vi "1_2_VisualAD_Train_Eval_Investigate.vi"(0 "NNFE_Paths":T1={"CFG"=path "D:/Ngene/GitHub/deepltk_examples/3_Image_Processing/36_Anomaly_Detection/NNFE/WRN_50_2_2_L3/WRN_50_2_2_BBoneL3.cfg", "BIN"=path "D:/Ngene/GitHub/deepltk_examples/3_Image_Processing/36_Anomaly_Detection/NNFE/WRN_50_2_2_L3/WRN_50_2_2_BBoneL3.bin"}, 1 "Dest. Path":path=path "D:/working", 2 "Dataset_Path(Train)":path=path "D:/Ngene/GitHub/deepltk_examples/3_Image_Processing/36_Anomaly_Detection/Dataset/Cards_3OfSpades/train", 3 "Dataset_Path(Validation)":path=path "D:/Ngene/GitHub/deepltk_examples/3_Image_Processing/36_Anomaly_Detection/Dataset/Cards_3OfSpades/test", 4 "Ground_Truth_Folder_Path":path, 5 "error in":errorcluster, 6 "NNFE CFG":T7={"Name"="3OfSpades", "Layer_Selection_By"=enum."Stride", "Feature_Layers"={"[LayerID, PatchSize]"=[{"Layer_ID"=4, "Patch_Size"=3}, {"Layer_ID"=16, "Patch_Size"=5}]}, "Interpolation_Type"=enum."Bi-Linear"}, 7 "Dim_Reduction":T11={"Method"=enum."Rnd_Proj", "Target_Dim"=300, "Seed"=42}, 8 "NNPC_Setup":T2={"Input_Dims"={"C"=3, "H"=320, "W"=272}, "mBatch"=1, "Device"=enum."GPU", "GPU Id"=0}, 9 "CoreSet_Params":T5={"Distance_Metric"=enum."Euclidean", "CoreSet_Size"=10000.0, "Start_idx"=3}) -> (11 "MemBank Size":i32=10000, 13 "dT_Total":dbl=8.99153380000007 format="%.2f", 14 "Model Paths":T1={"CFG"=path "D:/working/NNPC_3OfSpades.cfg", "BIN"=path "D:/working/NNPC_3OfSpades.bin"}, 15 "Evaluation Metrics":T13={"Evaluation_Metrics(Pixel)"={"Scores(Good)"={"X Values"=[2.1673927682638165, 2.522966259121895, 2.8785397499799728, 3.2341132408380506, 3.589686731696129, 3.945260222554207, 4.300833713412285, 4.656407204270362, 5.011980695128441, 5.367554185986519, 5.723127676844596, 6.078701167702675, 6.434274658560753, 6.78984814941883, 7.145421640276909, 7.500995131134987, 7.856568621993065, 8.212142112851144, 8.567715603709221, 8.923289094567298, 9.278862585425376, 9.634436076283453, 9.990009567141533, 10.345583057999612, 10.70115654885769, 11.056730039715767, 11.412303530573844, 11.767877021431921, 12.12345051229, 12.479024003148078, 12.834597494006157, 13.190170984864235, 13.545744475722312, 13.90131796658039, 14.256891457438469, 14.612464948296546, 14.968038439154626, 15.323611930012703, 15.67918542087078, 16.034758911728858, 16.390332402586935, 16.745905893445013, 17.10147938430309, 17.457052875161168, 17.81262636601925, 18.168199856877326, 18.523773347735403, 18.879346838593484, 19.234920329451562, 19.59049382030964, 19.946067311167717, 20.301640802025794, 20.65721429288387, 21.01278778374195, 21.368361274600026, 21.723934765458107, 22.079508256316185, 22.435081747174262, 22.79065523803234, 23.146228728890417, 23.501802219748498, 23.857375710606576, 24.212949201464653, 24.56852269232273, 24.924096183180808, 25.279669674038885, 25.635243164896963, 25.99081665575504, 26.34639014661312, 26.7019636374712, 27.057537128329276, 27.413110619187353, 27.76868411004543, 28.124257600903512, 28.47983109176159, 28.835404582619667, 29.190978073477744, 29.54655156433582, 29.9021250551939, 30.257698546051977, 30.613272036910054, 30.968845527768135, 31.324419018626212, 31.67999250948429, 32.035566000342364, 32.39113949120044, 32.746712982058526, 33.1022864729166, 33.45785996377468, 33.81343345463276, 34.169006945490835, 34.52458043634891, 34.88015392720699, 35.23572741806507, 35.591300908923145, 35.94687439978122, 36.30244789063931, 36.658021381497385, 37.01359487235546, 37.36916836321354], "Histogram: h(x)"=[1, 13, 52, 84, 115, 188, 266, 742, 1993, 4173, 6263, 6873, 6767, 7084, 7294, 7385, 7892, 8253, 8640, 10003, 11295, 15100, 22306, 35779, 62043, 98920, 135969, 166467, 171557, 159572, 143358, 124535, 97728, 76352, 57016, 39265, 26147, 16432, 10767, 6225, 3406, 1671, 480, 165, 84, 0, 0, 0, 0, 0, 0, 0, 0, 0, 0, 0, 0, 0, 0, 0, 0, 0, 0, 0, 0, 0, 0, 0, 0, 0, 0, 0, 0, 0, 0, 0, 0, 0, 0, 0, 0, 0, 0, 0, 0, 0, 0, 0, 0, 0, 0, 0, 0, 0, 0, 0, 0, 0, 0, 0]}, "Scores(Bad)"={"X Values"=[2.1673927682638165, 2.522966259121895, 2.8785397499799728, 3.2341132408380506, 3.589686731696129, 3.945260222554207, 4.300833713412285, 4.656407204270362, 5.011980695128441, 5.367554185986519, 5.723127676844596, 6.078701167702675, 6.434274658560753, 6.78984814941883, 7.145421640276909, 7.500995131134987, 7.856568621993065, 8.212142112851144, 8.567715603709221, 8.923289094567298, 9.278862585425376, 9.634436076283453, 9.990009567141533, 10.345583057999612, 10.70115654885769, 11.056730039715767, 11.412303530573844, 11.767877021431921, 12.12345051229, 12.479024003148078, 12.834597494006157, 13.190170984864235, 13.545744475722312, 13.90131796658039, 14.256891457438469, 14.612464948296546, 14.968038439154626, 15.323611930012703, 15.67918542087078, 16.034758911728858, 16.390332402586935, 16.745905893445013, 17.10147938430309, 17.457052875161168, 17.81262636601925, 18.168199856877326, 18.523773347735403, 18.879346838593484, 19.234920329451562, 19.59049382030964, 19.946067311167717, 20.301640802025794, 20.65721429288387, 21.01278778374195, 21.368361274600026, 21.723934765458107, 22.079508256316185, 22.435081747174262, 22.79065523803234, 23.146228728890417, 23.501802219748498, 23.857375710606576, 24.212949201464653, 24.56852269232273, 24.924096183180808, 25.279669674038885, 25.635243164896963, 25.99081665575504, 26.34639014661312, 26.7019636374712, 27.057537128329276, 27.413110619187353, 27.76868411004543, 28.124257600903512, 28.47983109176159, 28.835404582619667, 29.190978073477744, 29.54655156433582, 29.9021250551939, 30.257698546051977, 30.613272036910054, 30.968845527768135, 31.324419018626212, 31.67999250948429, 32.035566000342364, 32.39113949120044, 32.746712982058526, 33.1022864729166, 33.45785996377468, 33.81343345463276, 34.169006945490835, 34.52458043634891, 34.88015392720699, 35.23572741806507, 35.591300908923145, 35.94687439978122, 36.30244789063931, 36.658021381497385, 37.01359487235546, 37.36916836321354], "Histogram: h(x)"=[8, 31, 105, 130, 214, 331, 610, 1315, 3212, 6453, 8836, 10903, 11627, 10731, 11893, 12681, 12586, 13151, 14679, 16111, 18152, 22770, 29905, 42923, 63976, 97131, 135040, 170047, 186000, 191189, 185809, 165467, 145942, 127004, 108579, 95369, 82034, 66973, 56446, 48734, 41993, 35860, 33251, 29363, 25936, 23587, 20606, 18581, 16403, 14613, 12756, 11558, 10975, 10578, 9887, 8831, 9074, 8615, 7970, 7376, 6857, 6950, 6755, 6391, 5609, 4681, 3976, 3457, 3231, 2862, 2517, 2294, 2141, 1977, 1864, 1796, 1866, 1798, 1579, 1481, 1246, 1074, 1034, 809, 645, 542, 391, 316, 340, 331, 318, 257, 219, 149, 152, 115, 99, 73, 53, 45]}, "Eval Stats"={"Scores(Good)"={"Min"=2.329183, "Max"=17.973423}, "Scores(Bad)"={"Min"=1.989606, "Max"=37.546955}, "# of Samples(Good)"=1566720, "# of Samples(Bad)"=2611200, "AUROC"=-1.0, "F1_Max"=-1.0, "Thrshld(F1_Max)"=17.973423, "Prec.(F1_Max)"=-1.0, "Recall(F1_Max)"=-1.0, "FPR(F1_Max)"=-1.0, "FNR(F1_Max)"=-1.0}}, "Evaluation_Metrics(Image)"={"Scores(Good)"={"X Values"=[16.63672716140747, 16.8714089012146, 17.10609064102173, 17.34077238082886, 17.575454120635985, 17.810135860443115, 18.044817600250244, 18.279499340057374, 18.514181079864503, 18.74886281967163, 18.98354455947876, 19.218226299285888, 19.452908039093018, 19.687589778900147, 19.922271518707277, 20.156953258514406, 20.391634998321535, 20.62631673812866, 20.86099847793579, 21.09568021774292, 21.33036195755005, 21.565043697357176, 21.799725437164305, 22.034407176971435, 22.269088916778564, 22.503770656585694, 22.738452396392823, 22.973134136199953, 23.207815876007082, 23.44249761581421, 23.677179355621337, 23.911861095428467, 24.146542835235596, 24.381224575042726, 24.615906314849852, 24.85058805465698, 25.08526979446411, 25.31995153427124, 25.55463327407837, 25.7893150138855, 26.02399675369263, 26.258678493499758, 26.493360233306888, 26.728041973114017, 26.962723712921143, 27.197405452728272, 27.4320871925354, 27.666768932342528, 27.901450672149657, 28.136132411956787, 28.370814151763916, 28.605495891571046, 28.840177631378175, 29.074859371185305, 29.309541110992434, 29.544222850799564, 29.77890459060669, 30.01358633041382, 30.24826807022095, 30.482949810028074, 30.717631549835204, 30.952313289642333, 31.186995029449463, 31.421676769256592, 31.656358509063722, 31.89104024887085, 32.12572198867798, 32.36040372848511, 32.59508546829224, 32.82976720809936, 33.06444894790649, 33.29913068771362, 33.53381242752075, 33.76849416732788, 34.00317590713501, 34.23785764694214, 34.47253938674927, 34.7072211265564, 34.94190286636353, 35.17658460617066, 35.411266345977786, 35.645948085784916, 35.880629825592045, 36.115311565399175, 36.349993305206304, 36.584675045013434, 36.819356784820556, 37.054038524627686, 37.288720264434815, 37.523402004241944, 37.758083744049074, 37.9927654838562, 38.22744722366333, 38.462128963470455, 38.696810703277585, 38.931492443084714, 39.166174182891844, 39.40085592269897, 39.6355376625061, 39.87021940231323], "Histogram: h(x)"=[2, 0, 0, 1, 2, 0, 1, 2, 3, 3, 2, 1, 0, 0, 1, 0, 0, 0, 0, 0, 0, 0, 0, 0, 0, 0, 0, 0, 0, 0, 0, 0, 0, 0, 0, 0, 0, 0, 0, 0, 0, 0, 0, 0, 0, 0, 0, 0, 0, 0, 0, 0, 0, 0, 0, 0, 0, 0, 0, 0, 0, 0, 0, 0, 0, 0, 0, 0, 0, 0, 0, 0, 0, 0, 0, 0, 0, 0, 0, 0, 0, 0, 0, 0, 0, 0, 0, 0, 0, 0, 0, 0, 0, 0, 0, 0, 0, 0, 0, 0]}, "Scores(Bad)"={"X Values"=[16.63672716140747, 16.8714089012146, 17.10609064102173, 17.34077238082886, 17.575454120635985, 17.810135860443115, 18.044817600250244, 18.279499340057374, 18.514181079864503, 18.74886281967163, 18.98354455947876, 19.218226299285888, 19.452908039093018, 19.687589778900147, 19.922271518707277, 20.156953258514406, 20.391634998321535, 20.62631673812866, 20.86099847793579, 21.09568021774292, 21.33036195755005, 21.565043697357176, 21.799725437164305, 22.034407176971435, 22.269088916778564, 22.503770656585694, 22.738452396392823, 22.973134136199953, 23.207815876007082, 23.44249761581421, 23.677179355621337, 23.911861095428467, 24.146542835235596, 24.381224575042726, 24.615906314849852, 24.85058805465698, 25.08526979446411, 25.31995153427124, 25.55463327407837, 25.7893150138855, 26.02399675369263, 26.258678493499758, 26.493360233306888, 26.728041973114017, 26.962723712921143, 27.197405452728272, 27.4320871925354, 27.666768932342528, 27.901450672149657, 28.136132411956787, 28.370814151763916, 28.605495891571046, 28.840177631378175, 29.074859371185305, 29.309541110992434, 29.544222850799564, 29.77890459060669, 30.01358633041382, 30.24826807022095, 30.482949810028074, 30.717631549835204, 30.952313289642333, 31.186995029449463, 31.421676769256592, 31.656358509063722, 31.89104024887085, 32.12572198867798, 32.36040372848511, 32.59508546829224, 32.82976720809936, 33.06444894790649, 33.29913068771362, 33.53381242752075, 33.76849416732788, 34.00317590713501, 34.23785764694214, 34.47253938674927, 34.7072211265564, 34.94190286636353, 35.17658460617066, 35.411266345977786, 35.645948085784916, 35.880629825592045, 36.115311565399175, 36.349993305206304, 36.584675045013434, 36.819356784820556, 37.054038524627686, 37.288720264434815, 37.523402004241944, 37.758083744049074, 37.9927654838562, 38.22744722366333, 38.462128963470455, 38.696810703277585, 38.931492443084714, 39.166174182891844, 39.40085592269897, 39.6355376625061, 39.87021940231323], "Histogram: h(x)"=[0, 0, 0, 0, 0, 0, 0, 0, 0, 0, 0, 0, 0, 0, 0, 0, 0, 0, 0, 0, 0, 1, 0, 0, 0, 1, 0, 0, 0, 0, 0, 1, 0, 0, 0, 0, 0, 0, 1, 0, 0, 1, 0, 0, 0, 0, 1, 0, 1, 0, 2, 2, 0, 0, 0, 1, 1, 1, 1, 0, 2, 2, 0, 0, 0, 0, 2, 0, 0, 1, 0, 0, 1, 1, 0, 0, 0, 0, 0, 0, 0, 1, 0, 0, 0, 0, 0, 0, 1, 0, 0, 0, 0, 0, 2, 1, 0, 0, 0, 1]}, "Eval Stats"={"Scores(Good)"={"Min"=16.519386, "Max"=19.817144}, "Scores(Bad)"={"Min"=21.46867, "Max"=39.98756}, "# of Samples(Good)"=18, "# of Samples(Bad)"=30, "AUROC"=1.0904129, "F1_Max"=-1.0, "Thrshld(F1_Max)"=20.642906, "Prec.(F1_Max)"=-1.0, "Recall(F1_Max)"=-1.0, "FPR(F1_Max)"=-1.0, "FNR(F1_Max)"=-1.0}}} {"Evaluation_Metrics(Image)"."Eval Stats"."Recall(F1_Max)" format="%#.5f"; "Evaluation_Metrics(Image)"."Eval Stats"."FPR(F1_Max)" format="%#.5f"; "Evaluation_Metrics(Image)"."Eval Stats"."FNR(F1_Max)" format="%#.5f"; "Evaluation_Metrics(Image)"."Eval Stats"."Prec.(F1_Max)" format="%#.5f"; "Evaluation_Metrics(Image)"."Eval Stats"."F1_Max" format="%#.5f"; "Evaluation_Metrics(Image)"."Eval Stats"."AUROC" format="%#.5f"; "Evaluation_Metrics(Image)"."Eval Stats"."Scores(Bad)"."Min" format="%#_5g"; "Evaluation_Metrics(Image)"."Eval Stats"."Scores(Good)"."Min" format="%#_5g"; "Evaluation_Metrics(Image)"."Eval Stats"."Thrshld(F1_Max)" format="%#_5f"; "Evaluation_Metrics(Pixel)"."Eval Stats"."Recall(F1_Max)" format="%#.5f"; "Evaluation_Metrics(Pixel)"."Eval Stats"."FPR(F1_Max)" format="%#.5f"; "Evaluation_Metrics(Pixel)"."Eval Stats"."FNR(F1_Max)" format="%#.5f"; "Evaluation_Metrics(Pixel)"."Eval Stats"."Prec.(F1_Max)" format="%#.5f"; "Evaluation_Metrics(Pixel)"."Eval Stats"."F1_Max" format="%#.5f"; "Evaluation_Metrics(Pixel)"."Eval Stats"."AUROC" format="%#.5f"; "Evaluation_Metrics(Pixel)"."Eval Stats"."Scores(Bad)"."Min" format="%#_5g"; "Evaluation_Metrics(Pixel)"."Eval Stats"."Scores(Good)"."Min" format="%#_5g"; "Evaluation_Metrics(Pixel)"."Eval Stats"."Thrshld(F1_Max)" format="%#_5f"}, 18 "Dataset Size":i32=20)   [LabVIEW 2020]
uses:
  <vilib>/Ngene/DeepLTK Anomaly Detection Addon/Toolkit/API/Controls/NN_Paths.ctl
  <vilib>/Ngene/DeepLTK Anomaly Detection Addon/Toolkit/API/Controls/NNPC_Setup.ctl
  <vilib>/Ngene/Deep Learning Toolkit/Toolkit/NN_Data/API/NN_Dims(C,H,W).ctl
  <vilib>/Ngene/Deep Learning Toolkit/Toolkit/NN_Network/Controls/NN_Device.ctl
  <vilib>/Ngene/DeepLTK Anomaly Detection Addon/Toolkit/API/Controls/NNPC_Coreset_Params.ctl
  <vilib>/Ngene/DeepLTK Anomaly Detection Addon/Toolkit/API/Controls/Distance_Metric.ctl
  <vilib>/Ngene/DeepLTK Anomaly Detection Addon/Toolkit/API/Controls/NNFE_CFG.ctl
  <vilib>/Ngene/DeepLTK Anomaly Detection Addon/Toolkit/API/Controls/Layer_Selector.ctl
  <vilib>/Ngene/DeepLTK Anomaly Detection Addon/Toolkit/API/Controls/Feature_Layer_Selector.ctl
  <vilib>/Ngene/DeepLTK Anomaly Detection Addon/Toolkit/API/Controls/Interpolation_Selector.ctl
  <vilib>/Ngene/DeepLTK Anomaly Detection Addon/Toolkit/API/Controls/NNPC_Random_Projection_CFG.ctl
  <vilib>/Ngene/DeepLTK Anomaly Detection Addon/Toolkit/API/Controls/Dim_Reduction_Method.ctl
  <vilib>/Ngene/DeepLTK Anomaly Detection Addon/Toolkit/API/Controls/Evaluation_Metrics(Pixel_Image).ctl
  <vilib>/Ngene/DeepLTK Anomaly Detection Addon/Toolkit/API/Controls/Evaluation_Metrics.ctl
  <vilib>/Ngene/DeepLTK Anomaly Detection Addon/Toolkit/API/Controls/Eval_Results.ctl
  <vilib>/Ngene/DeepLTK Anomaly Detection Addon/Toolkit/API/Controls/MinMax.ctl
  subVIs/Feature_Retrieval/Controls/Patch_RF_Scales.ctl
  subVIs/Dataset_Reader/Controls/Read_Options.ctl
  <vilib>/Ngene/DeepLTK Anomaly Detection Addon/Toolkit/API/Controls/NNPC_PreProcessing_Options.ctl
  <vilib>/Ngene/DeepLTK Anomaly Detection Addon/Toolkit/API/Controls/Crop_CFG.ctl
  <vilib>/Ngene/DeepLTK Anomaly Detection Addon/Toolkit/API/Controls/NNPC_DS_Stats.ctl
  <vilib>/Ngene/DeepLTK Anomaly Detection Addon/Toolkit/API/Controls/Image_Stats_RGB.ctl
  subVIs/Train_Case_Investigation/Controls/Detection_Results.ctl
  <vilib>/Ngene/DeepLTK Anomaly Detection Addon/Toolkit/API/Controls/Feature_Scorer_Params.ctl
  <vilib>/Ngene/DeepLTK Anomaly Detection Addon/Toolkit/API/Controls/Gaussian_Blur.ctl
  <vilib>/vision/Image Controls.llb/IMAQ Image.ctl
  subVIs/Visualizer/Controls/Display_Options.ctl
  subVIs/Visualizer/Controls/ROI_Display_Options.ctl
  subVIs/Visualizer/Controls/Heatmap_Display_Options.ctl
  subVIs/Visualizer/Controls/ColorMap.ctl
  subVIs/Visualizer/Controls/Report_Images_CFG.ctl
  <vilib>/Ngene/CuLab - GPU Accelerated Toolkit/Toolkit/Low_Level/Tensor_Classes/T_Children/T2D/T2D_Children/T2D_SGL/T2D_SGL.lvclass
  subVIs/Feature_Retrieval/Controls/Dims(2D)ctl.ctl
  4cc6689b-300a-41eb-b37a-9ba3a5a9262f.vi
  f46c6ce4-2999-47cd-b61f-bf4da423de8f.vi
  <vilib>/Utility/High Resolution Relative Seconds.vi
  <vilib>/Ngene/DeepLTK Anomaly Detection Addon/Toolkit/API/NNPC_Predict/NNPC_Predict(Dataset).vi
  <vilib>/Ngene/DeepLTK Anomaly Detection Addon/Toolkit/API/NNPC_Predict/NNPC_Predict(Single).vi
  <vilib>/Ngene/Deep Learning Toolkit/Toolkit/NN_Data/subVIs/Get_Data_Vals/2D/NN_Data_Get_ValByRef(2D_SGL).vi
  <vilib>/Ngene/CuLab - GPU Accelerated Toolkit/Toolkit/Low_Level/Tensor_Classes/T_Children/T2D/T2D_Children/T2D_SGL/Pull.vi
  <vilib>/Ngene/DeepLTK Anomaly Detection Addon/Toolkit/DeepLTK_Anomaly_Detection_Addon.lvlib
  <vilib>/Ngene/Deep Learning Toolkit/Toolkit/Deep_Learning_Toolkit_by_Ngene.lvlib
  <vilib>/Ngene/CuLab - GPU Accelerated Toolkit/Toolkit/CuLab.lvlib
  <vilib>/ptbypt/NI_PtbyPt.lvlib
  <vilib>/vision/NI_Vision_Development_Module.lvlib
panel:
  out "Last Mouse Position:All Elements":cluster{"X":i32, "Y":i32}={"X"=128, "Y"=172}
  in  "?":enum32{"Train Eval", "Investigation"}(tab)
  out "dT_Gen_Embed":dbl=0.16472169999997277 format="%.2f"
  out "dT_Coreset":dbl=4.406857699999819 format="%.2f"
  out "Coreset_Max_Distances":sgl[](graph)
  out "dT_NN_Init":dbl=2.5163400999999794 format="%.2f"
  out "dT_Read_DS(Train)":dbl=0.30830639999976484 format="%.2f"
  out "dT_Read_DS(Test)":dbl=0.43927769999982047 format="%.2f"
  out "dT_Eval":dbl=0.9348227000000406 format="%.2f"
  out "dT_Predict(DS)":dbl=0.6623571000000084 format="%.2f"
  out "Coreset Max":sgl=72.34939
  out "Feature Size":i32=300
  out "Coreset Min":sgl=12.7185
  in  "Online_Coreset_Params":T5={"Distance_Metric"=enum."Euclidean", "CoreSet_Size"=-1.0, "Start_idx"=3}
  out "Closest_Train_Sample":T17(plugin-control)
  in  "UpScale Factor":sgl=1.0
  in  "index":i32=17 min=0 max=29
  out "Anomaly Detection Result":T17(plugin-control)
  out "Image_Thrshld (Eval)":sgl=20.6429
  in  "Image_Thrshld(Custom)":sgl=-1.0 format="%_5g"
  out "Pixel_Score(Max)":sgl=29.230766
  out "Image_File_Path":path=path "D:/Ngene/GitHub/deepltk_examples/3_Image_Processing/36_Anomaly_Detection/Dataset/Cards_3OfSpades/test/bad/bad_Cut_Twice_1967.bmp"
  out "Pixel_Thrshld (Eval)":sgl=17.9734
  out "Anomaly?":bool=TRUE
  out "Img_Score":sgl=30.951008
  in  "Pixel_Thrshld(Custom)":sgl=18.2 format="%_5g"
  in  "DS Selector":enum16{"Good", "Bad", "Both"}(ring)=enum."Bad"
  in  "Order":enum16{"Ascending", "Descending", "File"}(ring)
  out "error out":errorcluster
  in  "Closest_Idx":i32 min=0 max=3
  out "#Closest_Samples":i32=4
  in  "Feature Color":u32(colorbox)=2486016
  in  "ROI Scales":T18={"Receptive_Field"=1.0, "Patch"=1.0} {"Patch" min=0 max=0; "Receptive_Field" min=0 max=0}
  out "Closest_Score":sgl=15.526439
  in  "Show Patch Grid?":bool
  in  "Search Mode":bool
  in  "Heatmap Range":T16={"Min"=17.0, "Max"=19.0} {"Min" format="%#_5g"}
  in  "ROI Color":u32(colorbox)=16717824
  in  "Display_Image":T19(ring)=enum."HeatMap"
  out "dT_Predict":dbl=0.014165199999922606 format="%#_3p"
  in  "Stop":bool
  out "Closest_Train_File_Path":path=path "D:/Ngene/GitHub/deepltk_examples/3_Image_Processing/36_Anomaly_Detection/Dataset/Cards_3OfSpades/train/good_2169.bmp"
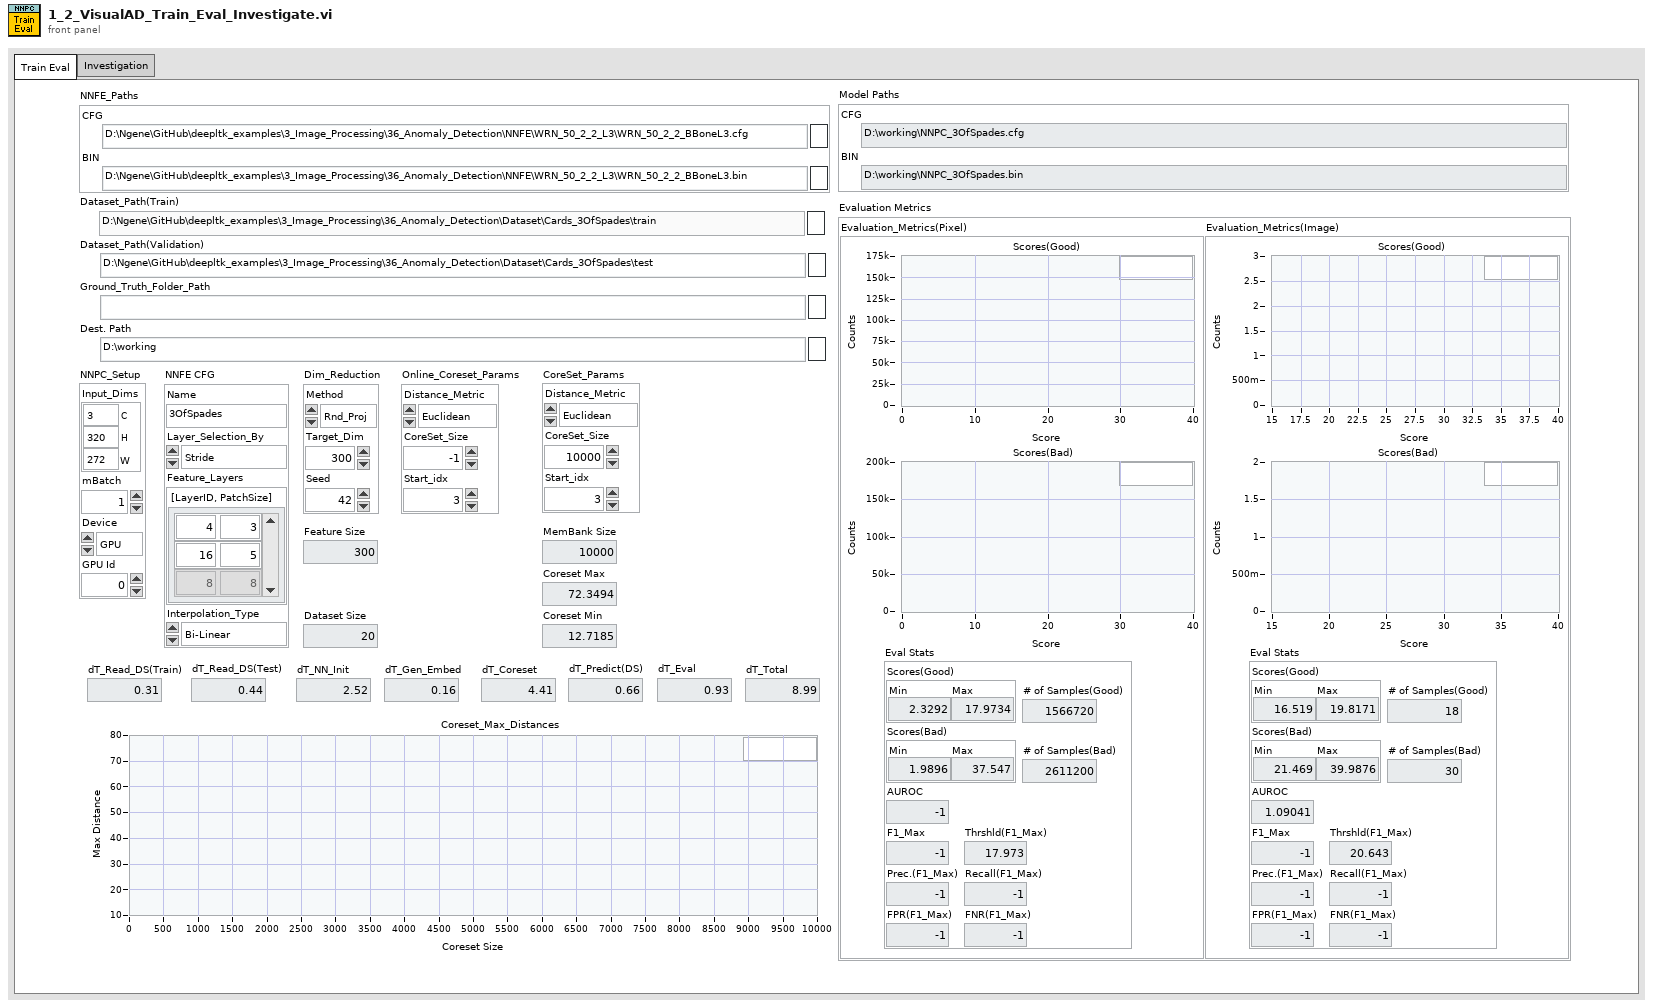
[diagram p1: front panel]
types:
  T1 = typedef "DeepLTK_Anomaly_Detection_Addon.lvlib/NN_Paths.ctl" = cluster{"CFG":path, "BIN":path}
  T2 = typedef "DeepLTK_Anomaly_Detection_Addon.lvlib/NNPC_Setup.ctl" = cluster{"Input_Dims":T3, "mBatch":i32, "Device":T4, "GPU Id":i32}
  T3 = typedef "Deep_Learning_Toolkit_by_Ngene.lvlib/NN_Dims(C,H,W).ctl" = cluster{"C":i32, "H":i32, "W":i32}
  T4 = typedef "Deep_Learning_Toolkit_by_Ngene.lvlib/NN_Device.ctl" = enum16{"CPU", "GPU"}
  T5 = typedef "DeepLTK_Anomaly_Detection_Addon.lvlib/NNPC_Coreset_Params.ctl" = cluster{"Distance_Metric":T6, "CoreSet_Size":sgl, "Start_idx":i32}
  T6 = typedef "DeepLTK_Anomaly_Detection_Addon.lvlib/Distance_Metric.ctl" = enum16{"Euclidean", "Cosine"}
  T7 = typedef "DeepLTK_Anomaly_Detection_Addon.lvlib/NNFE_CFG.ctl" = cluster{"Name":string, "Layer_Selection_By":T8, "Feature_Layers":T9, "Interpolation_Type":T10}
  T8 = typedef "DeepLTK_Anomaly_Detection_Addon.lvlib/Layer_Selector.ctl" = enum16{"Stride", "Layer_Idx"}
  T9 = typedef "DeepLTK_Anomaly_Detection_Addon.lvlib/Feature_Layer_Selector.ctl" = cluster{"[LayerID, PatchSize]":cluster{"Layer_ID":i32, "Patch_Size":i32}[]}
  T10 = typedef "DeepLTK_Anomaly_Detection_Addon.lvlib/Interpolation_Selector.ctl" = enum16{"Nearest", "Bi-Linear"}
  T11 = typedef "DeepLTK_Anomaly_Detection_Addon.lvlib/NNPC_Random_Projection_CFG.ctl" = cluster{"Method":T12, "Target_Dim":i32, "Seed":i32}
  T12 = typedef "DeepLTK_Anomaly_Detection_Addon.lvlib/Dim_Reduction_Method.ctl" = enum16{"None", "Rnd_Proj", "PCA"}
  T13 = typedef "DeepLTK_Anomaly_Detection_Addon.lvlib/Evaluation_Metrics(Pixel_Image).ctl" = cluster{"Evaluation_Metrics(Pixel)":T14, "Evaluation_Metrics(Image)":T14}
  T14 = typedef "DeepLTK_Anomaly_Detection_Addon.lvlib/Evaluation_Metrics.ctl" = cluster{"Scores(Good)":cluster{"X Values":dbl[], "Histogram: h(x)":i32[]}, "Scores(Bad)":cluster{"X Values":dbl[], "Histogram: h(x)":i32[]}, "Eval Stats":T15}
  T15 = typedef "DeepLTK_Anomaly_Detection_Addon.lvlib/Eval_Results.ctl" = cluster{"Scores(Good)":T16, "Scores(Bad)":T16, "# of Samples(Good)":i32, "# of Samples(Bad)":i32, "AUROC":sgl, "F1_Max":sgl, "Thrshld(F1_Max)":sgl, "Prec.(F1_Max)":sgl, "Recall(F1_Max)":sgl, "FPR(F1_Max)":sgl, "FNR(F1_Max)":sgl}
  T16 = typedef "DeepLTK_Anomaly_Detection_Addon.lvlib/MinMax.ctl" = cluster{"Min":sgl, "Max":sgl}
  T17 = typedef "IMAQ Image.ctl" = refnum<image>
  T18 = typedef "Patch_RF_Scales.ctl" = cluster{"Receptive_Field":sgl, "Patch":sgl}
  T19 = enum16{"Original", "Ground_Truth", "HeatMap", "Mask", "Segmentation"}
  T20 = typedef "Image Type" = u32
  T21 = typedef "DeepLTK_Anomaly_Detection_Addon.lvlib/Feature_Scorer_Params.ctl" = cluster{"Nearest_Neighbors":i32, "Calculate Anomaly Map":bool, "Gaussian_Blur":T22}
  T22 = typedef "DeepLTK_Anomaly_Detection_Addon.lvlib/Gaussian_Blur.ctl" = cluster{"Kernel_Size":i32, "Sigma":sgl}
  T23 = typedef "Detection_Results.ctl" = cluster{"Image Score":sgl, "Pixel Score":sgl[][], "File Path":path}
  T24 = typedef "Read_Options.ctl" = cluster{"Read Bads?":bool, "Read GTs?":bool, "Update. DS Stats?":bool}
  T25 = typedef "DeepLTK_Anomaly_Detection_Addon.lvlib/NNPC_PreProcessing_Options.ctl" = cluster{"DS_Name":string, "Input_Dims":T3, "Cropping":T26, "Interpolation Type":u32, "MultiStage_ReSample?":bool, "Dataset_Stats":T27}
  T26 = typedef "DeepLTK_Anomaly_Detection_Addon.lvlib/Crop_CFG.ctl" = cluster{"Left":sgl, "Top":sgl, "Right":sgl, "Bottom":sgl}
  T27 = typedef "DeepLTK_Anomaly_Detection_Addon.lvlib/NNPC_DS_Stats.ctl" = cluster{"means":T28, "stds":T28}
  T28 = typedef "DeepLTK_Anomaly_Detection_Addon.lvlib/Image_Stats_RGB.ctl" = cluster{"R":sgl, "G":sgl, "B":sgl}
  T29 = typedef "Deep_Learning_Toolkit_by_Ngene.lvlib/NN_DataSet(In3D_Out3D).ctl" = cluster{"Dataset_Size":i32, "Dims_In":T3, "Labels":string[], "File Paths":path[], "Outputs Ref.":T30, "Inputs Ref.":variant, "Dims_Out":T3, "Custom_Data":variant}
  T30 = typedef "Deep_Learning_Toolkit_by_Ngene.lvlib/NN_Data_ref(4D_SGL).ctl" = refnum<data-value>
  T31 = typedef "DeepLTK_Anomaly_Detection_Addon.lvlib/NNPC_Instance.ctl" = cluster{"Name":string, "NN":T32, "MemBank_Data":T46}
  T32 = typedef "Deep_Learning_Toolkit_by_Ngene.lvlib/NN.ctl" = cluster{"Name":string, "No of Layers":i32, "mBatch":i32, "Layers":T33[], "Dimty":T34, "Dims_In":T3, "Dims_Out":T3, "Working_Dir":path, "Train?":bool, "Train_Params":T35, "LR_Update_Policy":T38, "Session Data":T40, "Ground_truth":T41, "NNg_hdls":T42, "NN_Device":T4, "GPU Id":i32, "Labels":string[], "Loss_Type":T43, "Loss_Cfg_Prms":variant, "NNG_WS":T44, "DryRun?":bool}
  T33 = typedef "Deep_Learning_Toolkit_by_Ngene.lvlib/NN_Layer_ref.ctl" = refnum<file>
  T34 = typedef "Deep_Learning_Toolkit_by_Ngene.lvlib/NN_In_Out_Dim-ty.ctl" = enum8{"In1D_Out1D", "In3D_Out1D", "In3D_Out3D", "In3D_OutBBox"}
  T35 = typedef "Deep_Learning_Toolkit_by_Ngene.lvlib/NN_Train_Params.ctl" = cluster{"Optimizer":T36, "Beta_1":sgl, "Beta_2":sgl, "Weight Decay(L1)":sgl, "Weight Decay(L2)":sgl, "Data_Sampling":T37}
  T36 = typedef "Deep_Learning_Toolkit_by_Ngene.lvlib/NN_Train_Optimizer.ctl" = enum16{"SGD", "Adam", "Adagrad", "Adadelta", "RMSProp", "Nesterov"}
  T37 = typedef "Deep_Learning_Toolkit_by_Ngene.lvlib/NN_Train_Data_Sampling.ctl" = enum16{"Random", "Sequential"}
  T38 = typedef "Deep_Learning_Toolkit_by_Ngene.lvlib/NN_LR_Policy_Cfg.ctl" = cluster{"Policy_Type":T39, "LR0":dbl, "k":sgl, "WarmUp_Policy":enum16{"Step", "Ramp"}, "WarmUp_Iter":i32, "WarmUp_Ratio":sgl}
  T39 = typedef "Deep_Learning_Toolkit_by_Ngene.lvlib/NN_LR_Policy_Type.ctl" = enum16{"Manual", "Step", "Exp", "1/t"}
  T40 = typedef "Deep_Learning_Toolkit_by_Ngene.lvlib/NN_Train_Session_Data.ctl" = cluster{"Epochs":sgl, "Tot_Iter":i32, "LR":sgl, "LR_iter":i32}
  T41 = typedef "Deep_Learning_Toolkit_by_Ngene.lvlib/NN_Ground_truth.ctl" = cluster{"Y":variant}
  T42 = typedef "Deep_Learning_Toolkit_by_Ngene.lvlib/nng_cuda_handles.ctl" = cluster{"cudnn":u64, "cublas":u64, "stream":u64, "curand":u64}
  T43 = typedef "Deep_Learning_Toolkit_by_Ngene.lvlib/NN_Loss_Type.ctl" = enum16{"None", "MSE", "CrossEntropy", "YOLO_v2", "YOLO_v4"}
  T44 = typedef "Deep_Learning_Toolkit_by_Ngene.lvlib/NNG_WS.ctl" = cluster{"NNG_WS_Mem":T45, "Max_WS_Size":i64}
  T45 = typedef "Deep_Learning_Toolkit_by_Ngene.lvlib/NNg_WS_Mem_DVR.ctl" = refnum<data-value>
  T46 = typedef "DeepLTK_Anomaly_Detection_Addon.lvlib/MemBank_and_Norm_Variants.ctl" = cluster{"MemBank":variant, "MemBank Norm":variant}
  T47 = typedef "DeepLTK_Anomaly_Detection_Addon.lvlib/Feature_Coords(Idx,i,j).ctl" = cluster{"Idx":i32, "i":i32, "j":i32}
  T48 = typedef "imagedata.ctl" = cluster{"image type":i32, "image depth":i32, "image":u8[], "mask":u8[], "colors":u32[], "Rectangle":cluster{"left":i16, "top":i16, "right":i16, "bottom":i16}}
  T49 = typedef "DeepLTK_Anomaly_Detection_Addon.lvlib/NNPC_Evaluation_Results.ctl" = cluster{"Threshold(Image)":sgl, "Threshold(Pixel)":sgl, "Pixel_Range":cluster{"Min":sgl, "Max":sgl}}
  T50 = typedef "Selected_Coreset_Elements_and_Dim_Stride_Info.ctl" = cluster{"Dims_Out":T51, "Stride":i32, "Coreset_Elements":T47[]}
  T51 = typedef "Dims(2D)ctl.ctl" = cluster{"H":i32, "W":i32}
  T52 = typedef "Deep_Learning_Toolkit_by_Ngene.lvlib/NN_Layer.ctl" = cluster{"Name":string, "Layer_Data":T53, "Layer_Type":T54, "Dims_In":T3, "Layers_In":T33[], "Dims_Out":T3, "Layers_Out":T33[], "Metrics":T55, "GPU_Data":T56, "mBatch":i32, "NN_Device":T4, "NNg_hdls":T42, "Train?":bool, "Dimty":T57, "RecptField":T58, "Idx":i32}
  T53 = typedef "Deep_Learning_Toolkit_by_Ngene.lvlib/NN_Layer_Data_Refnum.ctl" = refnum<file>
  T54 = typedef "Deep_Learning_Toolkit_by_Ngene.lvlib/NN_Layer_Type.ctl" = enum16{"Input1D", "Input3D", "Conv1D", "Conv2D", "Conv2D_Adv", "MaxPool", "AvgPool", "UpSample", "DropOut3D", "ShortCut", "Concat", "SoftMax3D", "FC", "DropOut", "Softmax", "Flatten", "YOLO_v2", "YOLO_v4", "Activation", "BatchNormalization", "LayerNormalization", "Scale", "Unsupported"}
  T55 = typedef "Deep_Learning_Toolkit_by_Ngene.lvlib/NN_Layer_Metrics.ctl" = cluster{"Data":dbl, "Params":dbl, "Ops":dbl}
  T56 = typedef "Deep_Learning_Toolkit_by_Ngene.lvlib/NNg_Layer_Data_Refnum.ctl" = refnum<file>
  T57 = typedef "Deep_Learning_Toolkit_by_Ngene.lvlib/NN_Layer_Dimty.ctl" = enum16{"1D", "3D"}
  T58 = typedef "Deep_Learning_Toolkit_by_Ngene.lvlib/NN_Layer_RF_State.ctl" = cluster{"Dims":T59, "J":T59}
  T59 = typedef "Deep_Learning_Toolkit_by_Ngene.lvlib/NN_Dims(V,H).ctl" = cluster{"V":i32, "H":i32}
  T60 = typedef "Display_Options.ctl" = cluster{"ROI_Options":T61, "Heatmap_Options":T62, "Report_Images_CFG":T64}
  T61 = typedef "ROI_Display_Options.ctl" = cluster{"Color":u32, "Width":u32, "Drawing Mode":enum16{"Frame", "Fill"}}
  T62 = typedef "Heatmap_Display_Options.ctl" = cluster{"ColorMap":T63, "Alpha":sgl, "Heatmap Range":T16}
  T63 = typedef "ColorMap.ctl" = enum16{"Jet", "Perula", "Inferno", "Plasma", "Viridis"}
  T64 = typedef "Report_Images_CFG.ctl" = cluster{"Original Image":bool, "Ground Truth":bool, "HeatMap":bool, "Mask":bool, "Segmentation":bool}
  T65 = typedef "Anomaly_Detection_Results_Imgs.ctl" = cluster{"Image":T17, "Ground Truth":T17, "Predicted Heat Map":T17, "Predicted Mask":T17, "Segmentation":T17}
  T66 = typedef "Closest_Sample_Info.ctl" = cluster{"Score":sgl, "Feature_Coords":T47}
  T67 = typedef "Deep_Learning_Toolkit_by_Ngene.lvlib/NN_BBox.ctl" = cluster{"x":sgl, "y":sgl, "w":sgl, "h":sgl}
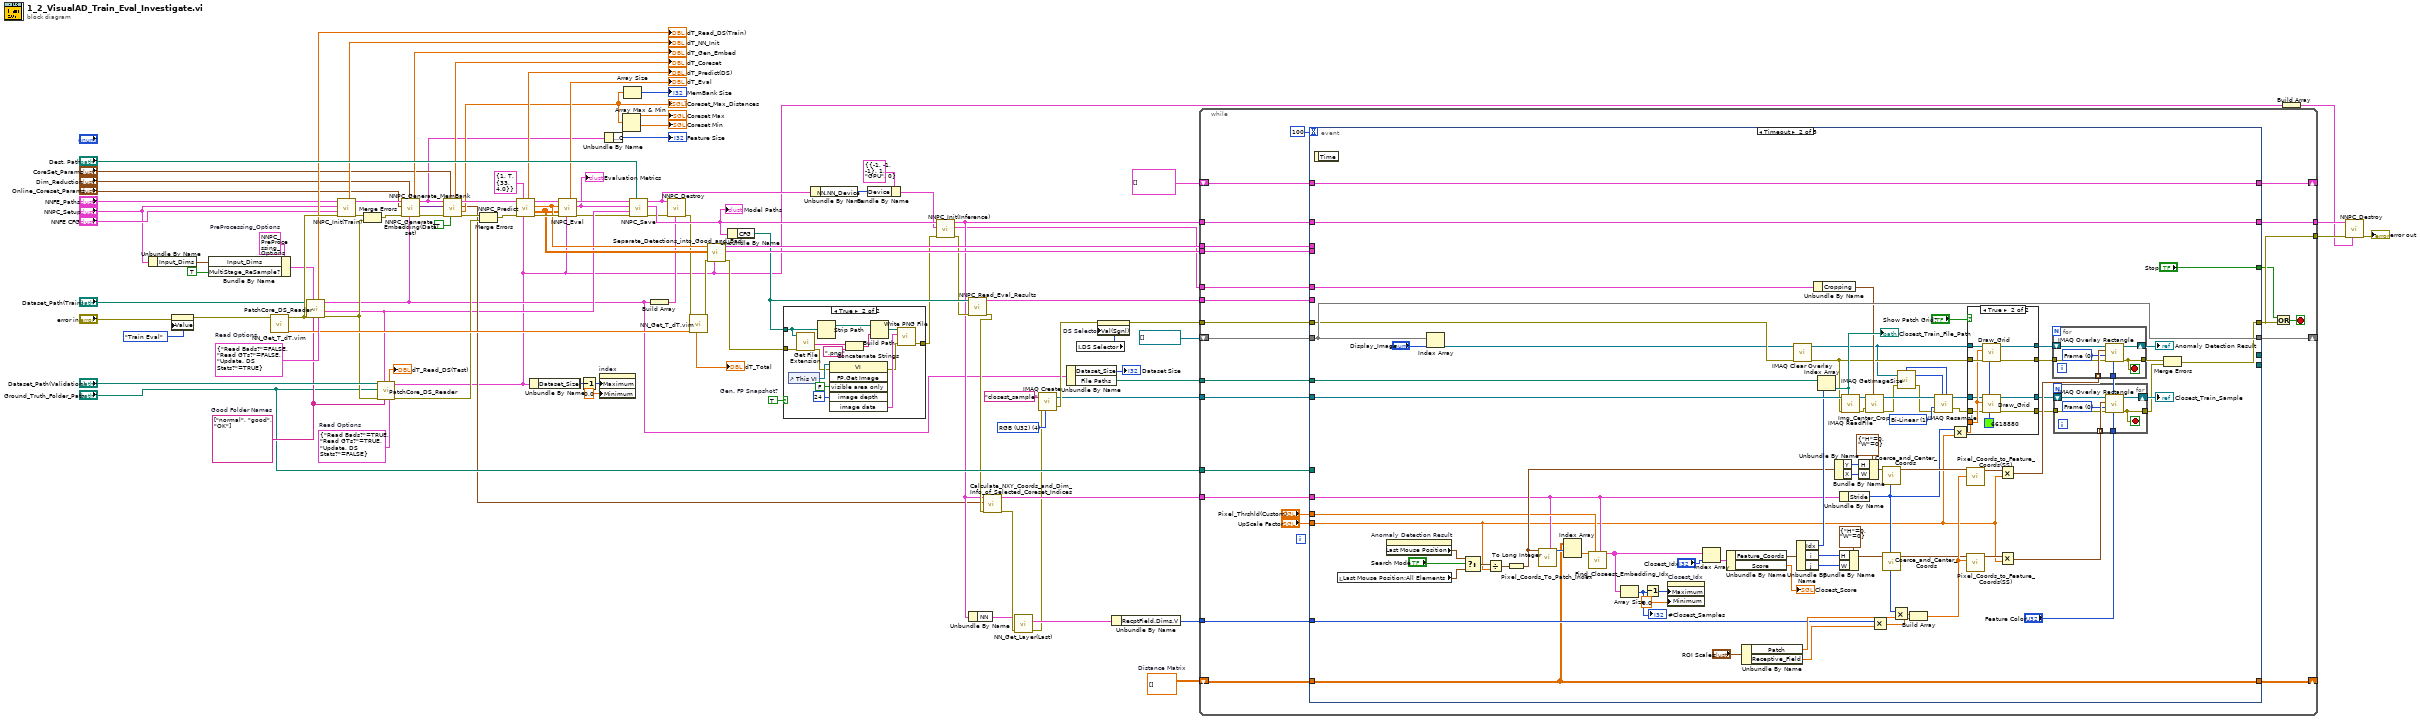
[diagram p0: block diagram]
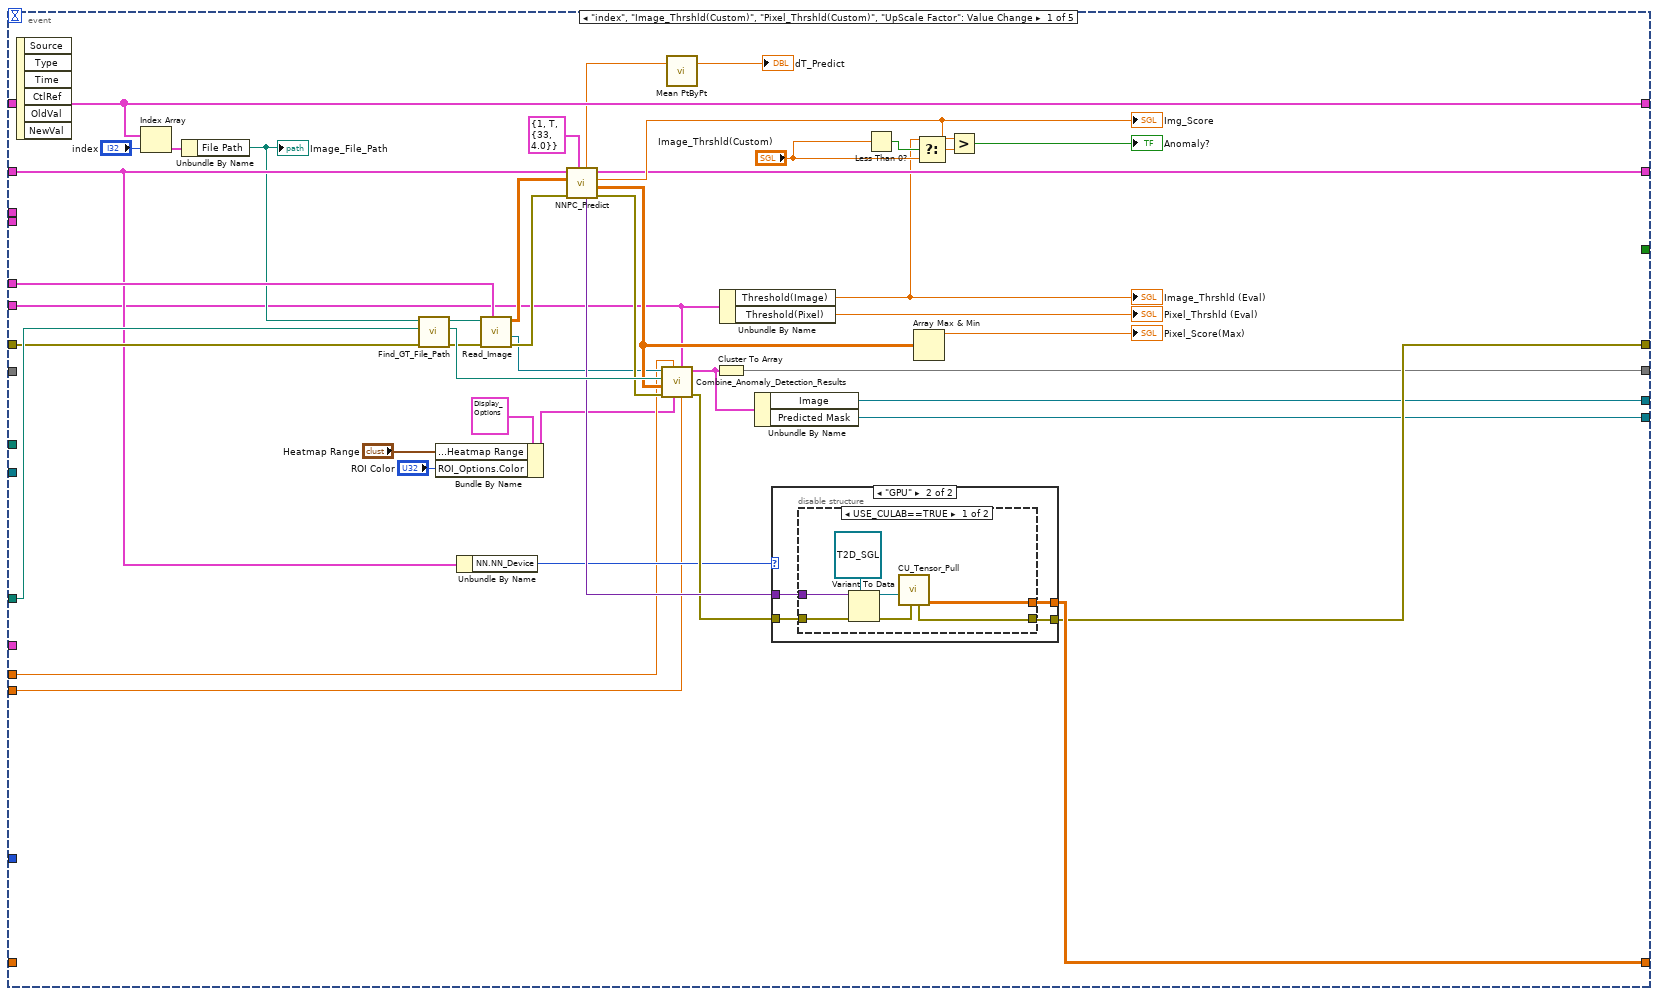
[diagram p2: hidden frame]
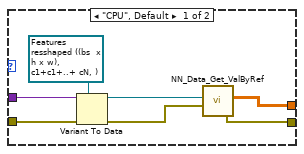
[diagram p3: hidden frame]
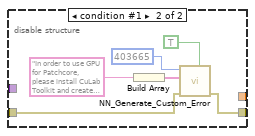
[diagram p4: hidden frame]
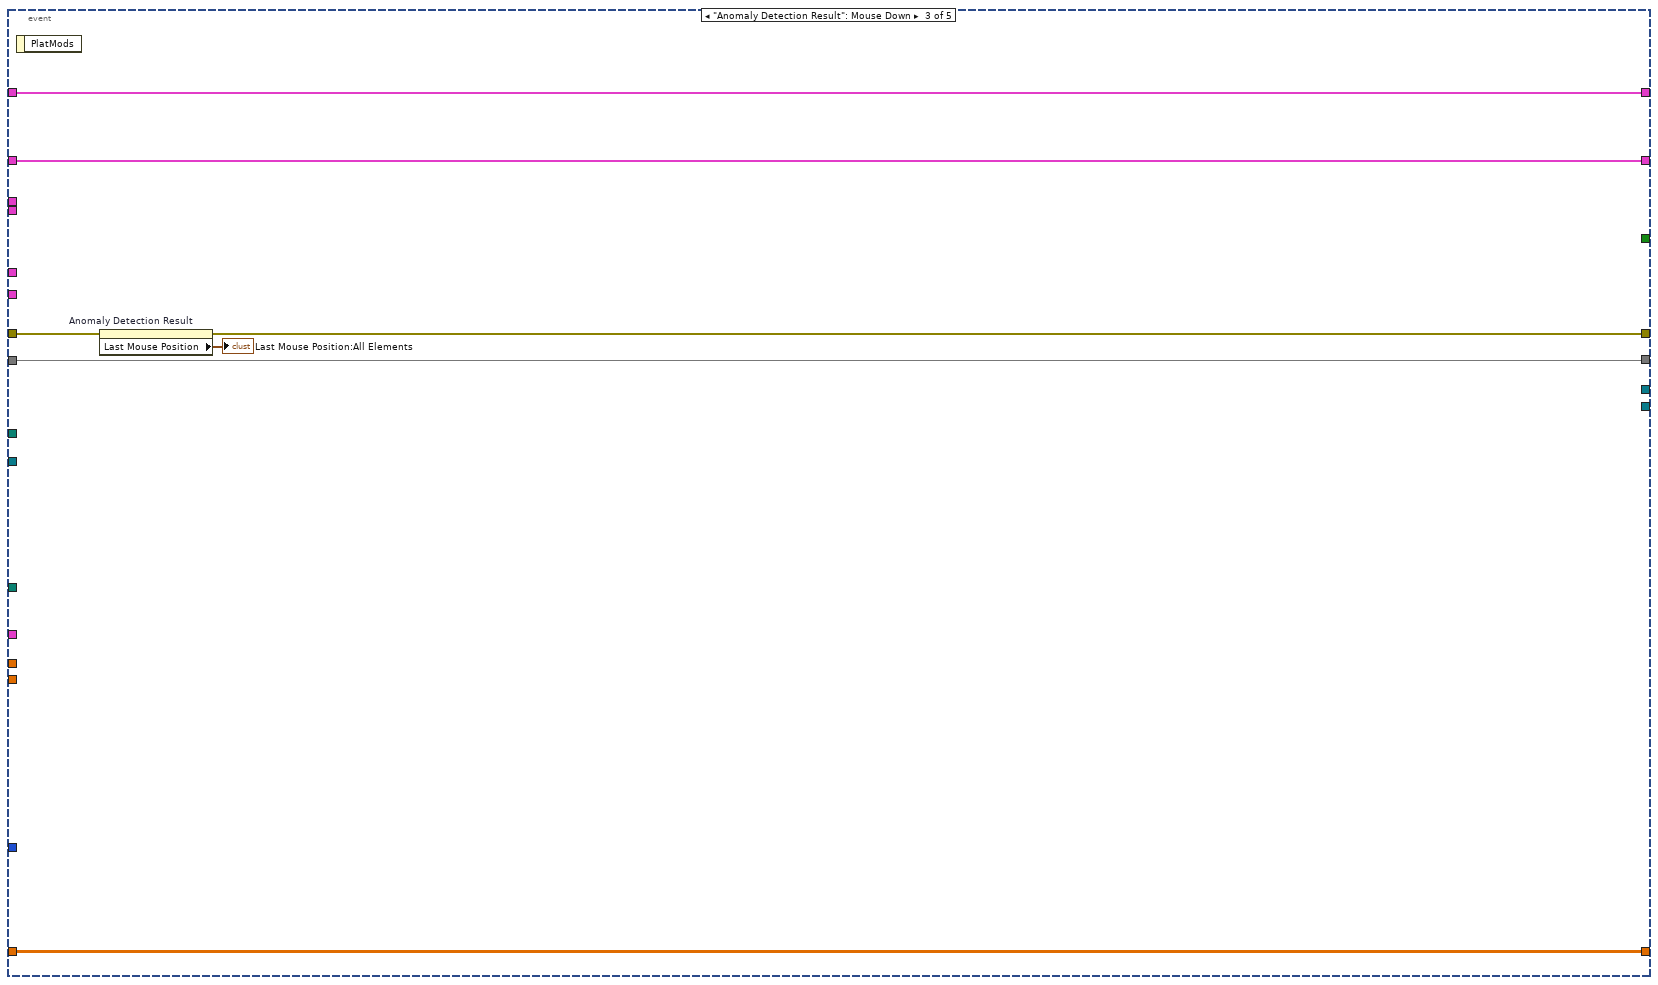
[diagram p6: hidden frame]
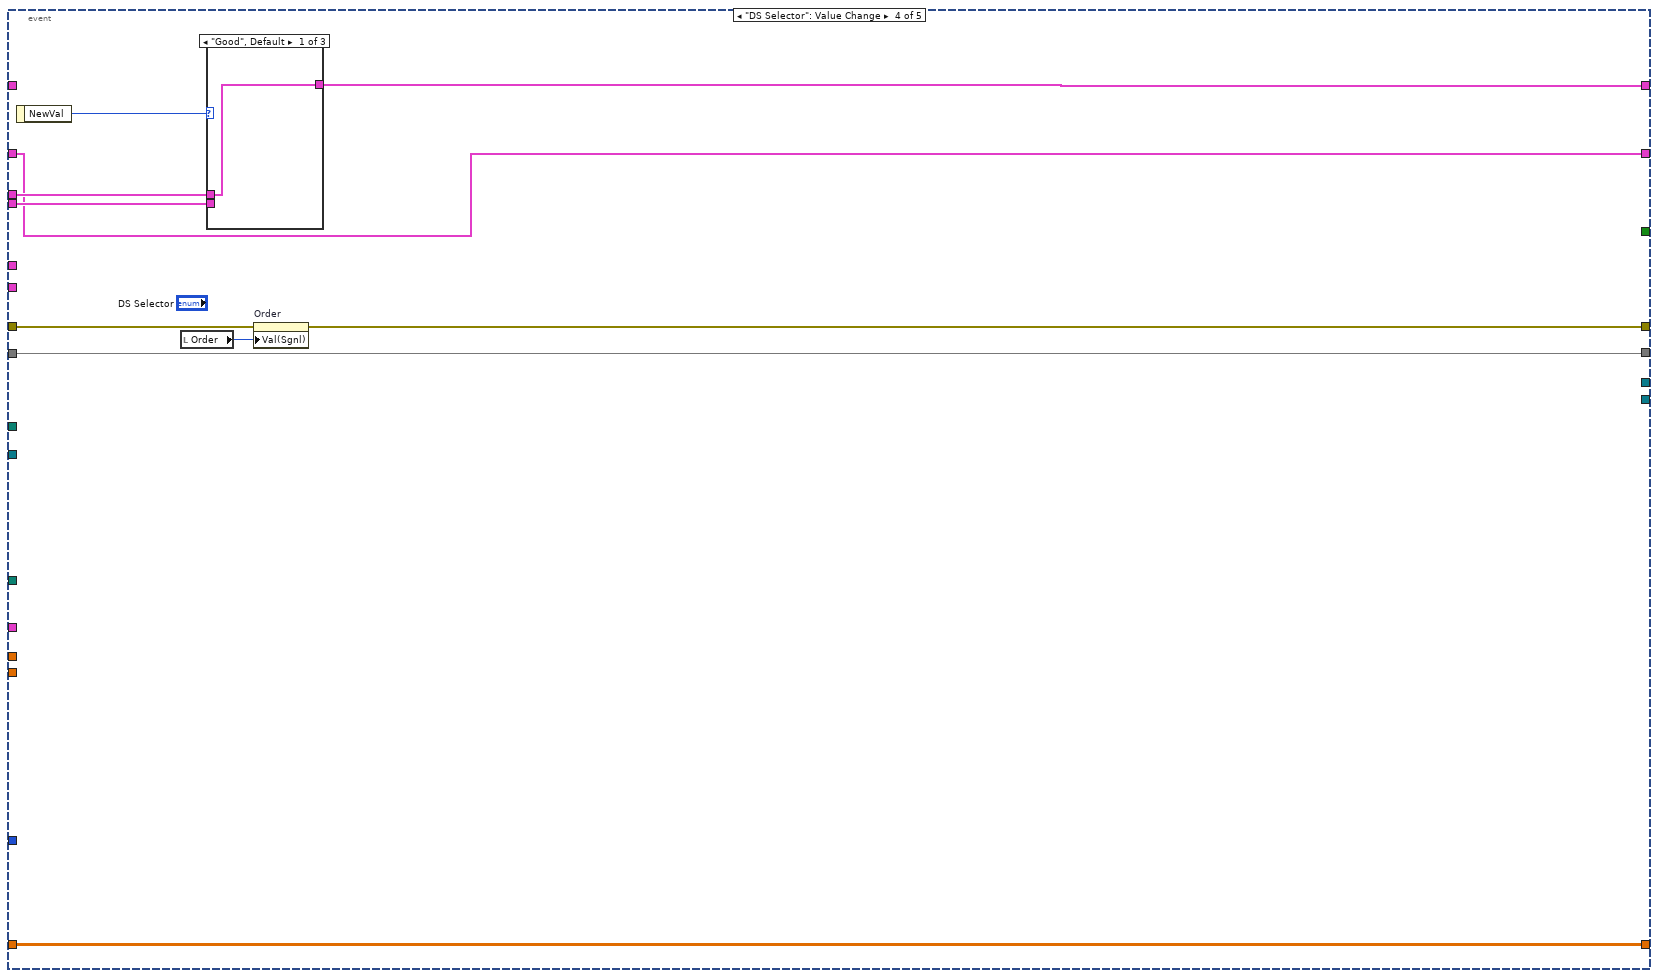
[diagram p7: hidden frame]
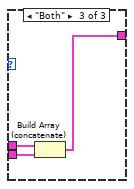
[diagram p9: hidden frame]
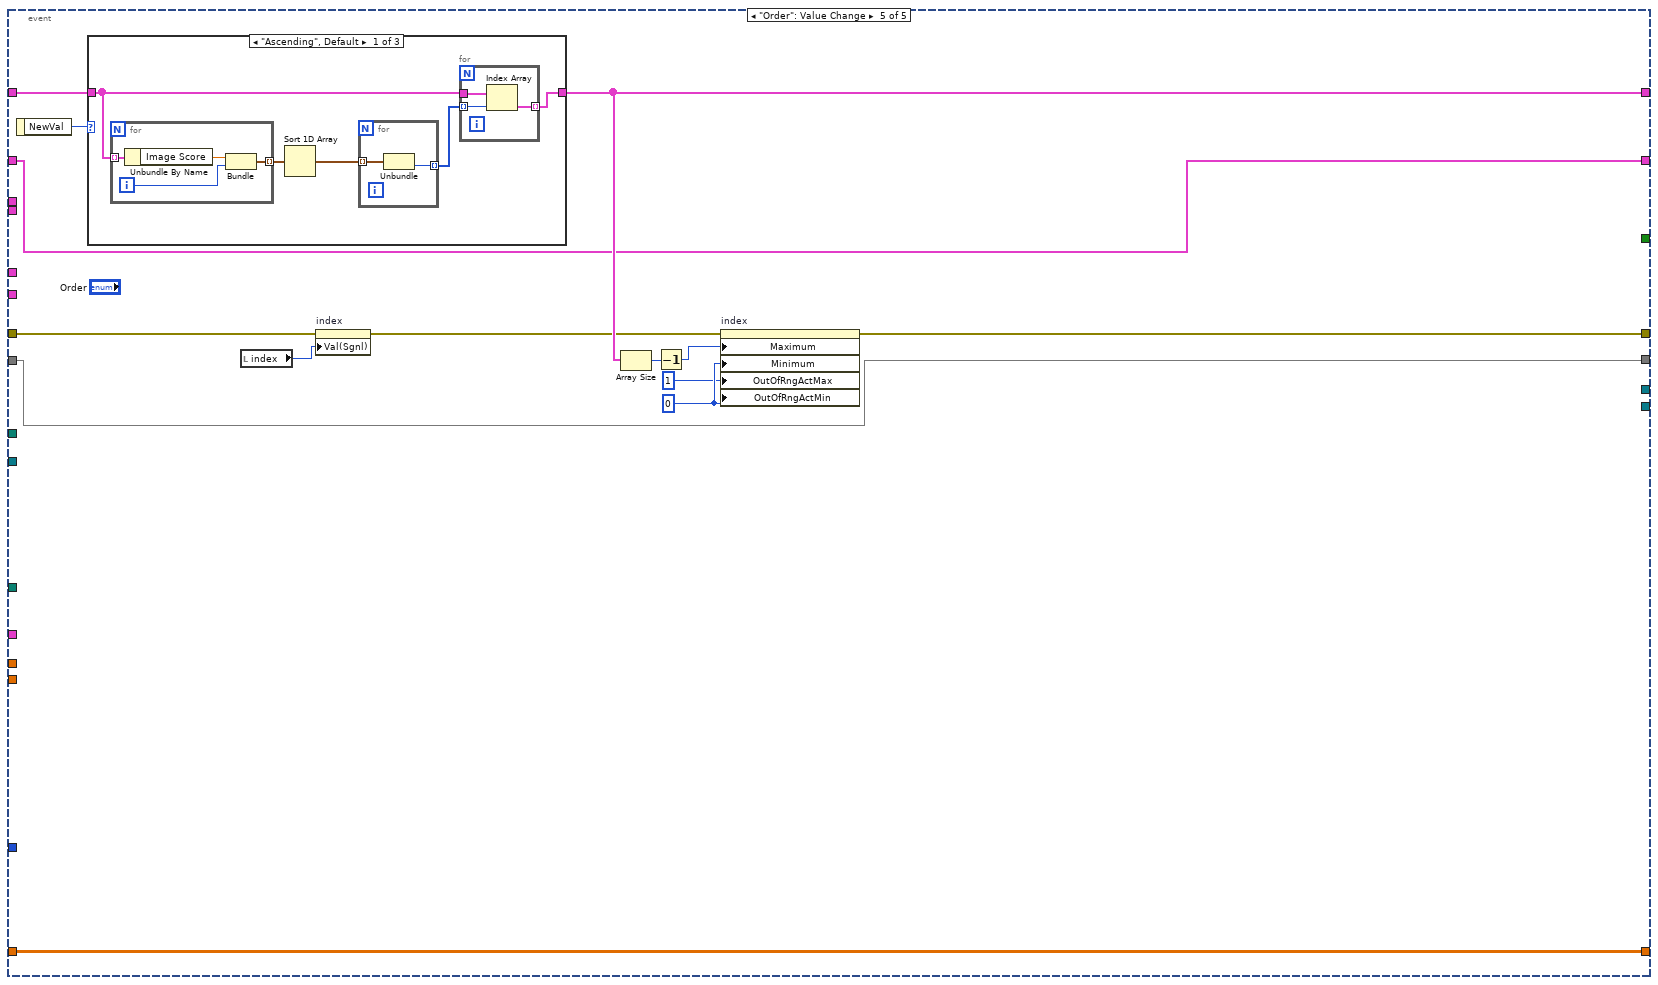
[diagram p10: hidden frame]
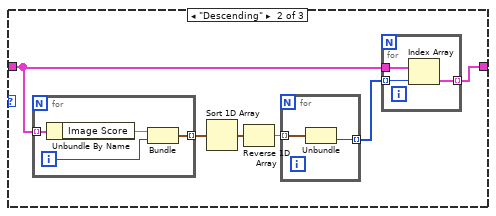
[diagram p11: hidden frame]
diagram:
  w36 = T20 4 items=["Grayscale (U8)", "Grayscale (I16)", "Grayscale (SGL)", "Complex (CSG)", "RGB (U32)", "HSL (U32)", "RGB (U64)", "Grayscale (U16)"] ("Image Type")
  w37 = sgl[][] []  # Distance Matrix
  w68 = TRUE  # Gen. FP Snapshot?
  w84 = T24 {"Read Bads?"=TRUE, "Read GTs?"=TRUE, "Update. DS Stats?"=FALSE}  # Read Options
  w95 = T25 {"DS_Name"="", "Input_Dims"={"C"=3, "H"=224, "W"=224}, "Cropping"={"Left"=0.0, "Top"=1.0, "Right"=0.0, "Bottom"=1.0}, "Interpolation Type"=1, "MultiStage_ReSample?"=FALSE, "Dataset_Stats"={"means"={"R"=0.0, "G"=0.0, "B"=0.0}, "stds"={"R"=1.0, "G"=1.0, "B"=1.0}}}  # PreProcessing_Options
  w92 = T24 {"Read Bads?"=FALSE, "Read GTs?"=FALSE, "Update. DS Stats?"=TRUE}  # Read Options
  w74 = string[] ["normal", "good", "OK"]  # Good Folder Names
  n1 = Unbundle By Name("NNPC_Setup") -> ("Input_Dims"=w93:T3)
  n2 = property class="TabCtl (strict)"(error in="error in", "Value"=enum32{"Train Eval", "Investigation"}."Train Eval") -> (error out=w60:errorcluster)  [unwired: 1 in, 1 out]
  n3 = Bundle By Name(cluster=w95, "Input_Dims"=w93, "MultiStage_ReSample?"=TRUE ("Multi-Stage_DownSample?")) -> (w52:T25)
  n4 = call "NN_Get_T_dT.vim"("error in"=w60) -> ("T_out"=w89:dbl, "error out"=w103:errorcluster)  [unwired: 6 in, 1 out]
  n5 = call "PatchCore_DS_Reader.vi"("Read Options"=w92, "Good Unique Labels"=w74, "PreProc_Options_in"=w52, "error in"=w103, "Folder Path"="Dataset_Path(Train)") -> ("error out"=w81:errorcluster, "PreProc_Options_out"=w13:T25, "Dataset"=w3:T29, "dT_DS_Reader"=→"dT_Read_DS(Train)":dbl)  [unwired: 3 in]
  n6 = call <vilib>:"NNPC_Init(Train).vi"("error in"=w103, "NNFE_CFG"="NNFE CFG", "NNPC_Setup"="NNPC_Setup", "NNFE_Paths"="NNFE_Paths") -> ("error out"=w99:errorcluster, "NNPC_out"=w98:T31, "dT_Init_Train"=→"dT_NN_Init":dbl)  [unwired: 5 in]
  n7 = Merge Errors(w99, w81) -> (w90:errorcluster)
  n8 = call "PatchCore_DS_Reader.vi"("Read Options"=w84, "Good Unique Labels"=w74, "PreProc_Options_in"=w13, "error in"=w81, "GT Folder Path"="Ground_Truth_Folder_Path", "Folder Path"="Dataset_Path(Validation)") -> ("error out"=w75:errorcluster, "Dataset"=w2:T29, "dT_DS_Reader"=→"dT_Read_DS(Test)":dbl)  [unwired: 2 in, 1 out]
  n9 = call <vilib>:"NNPC_Generate_Embedding(Dataset).vi"("Dataset"=w3, "Dim_Reduction"="Dim_Reduction", "error in"=w90, "Online_Coreset_Params"="Online_Coreset_Params", "NNPC_in"=w98) -> ("error out"=w28:errorcluster, "Feature_Embeddings"=w86:variant, "NNPC_out"=w53:T31, "dT_Embed"=→"dT_Gen_Embed":dbl)  [unwired: 2 in, 1 out]
  n10 = call <vilib>:"NNPC_Generate_MemBank.vi"("Destroy Embeds Afterwards?"=TRUE, "Coreset_Params"="CoreSet_Params", "error in"=w28, "Feature_Embeddings"=w86, "NNPC_in"=w53) -> ("error out"=w69:errorcluster, "Max_Distances"=w55:sgl[], "Selected_Feature_Coords"=w16:T47[], "NNPC_out"=w77:T31, "dT_Coreset"=→"dT_Coreset":dbl)  [unwired: 2 in]
  "Coreset_Max_Distances" <- w55
  n11 = Merge Errors(w69, w75) -> (w76:errorcluster)
  n12 = call-poly <vilib>:"NNPC_Predict.vi"("Dataset"=w2, "Feature_Scorer_Params"=T21 {"Nearest_Neighbors"=1, "Calculate Anomaly Map"=TRUE, "Gaussian_Blur"={"Kernel_Size"=33, "Sigma"=4.0}}, "error in"=w76, "NNPC_in"=w77) -> ("error out"=w78:errorcluster, "Anomaly_Maps"=w65:sgl[][][], "Pred_Scores"=w66:sgl[], "NNPC_out"=w73:T31, "dT_Predict"=→"dT_Predict(DS)":dbl)  [unwired: 3 in]
  n13 = Unbundle By Name(w2) -> ("Dataset_Size"=w46:i32)
  n14 = call <vilib>:"NNPC_Eval.vi"("Dataset"=w2, "error in"=w78, "Anomaly_Maps"=w65, "Pred_Scores"=w66, "NNPC_in"=w73) -> ("error out"=w9:errorcluster, "Evaluation_Metrics"=w4:T13, "NNPC_out"=w72:T31, "dT_Eval"=→"dT_Eval":dbl)  [unwired: 3 in]
  "Evaluation Metrics" <- w4
  n15 = Decrement(x=w46) -> (x-1=w48:i32)
  n16 = property on="index" class="DigNum (strict)"("Maximum"=w48, "Minimum"=0.0 ("Data Entry Limits:Minimum")) -> ()  [unwired: 2 in, 2 out]
  n17 = Unbundle By Name(w53) -> ("NN.Dims_Out.C"=→"Feature Size":i32)
  n18 = Array Max & Min(array=w55) -> (max value=→"Coreset Max":sgl, min value=→"Coreset Min":sgl)  [unwired: 2 out]
  n19 = Array Size(array=w55) -> (size(s)=→"MemBank Size":i32)
  n20 = call <vilib>:"NNPC_Save.vi"("Dst_Folder"="Dest. Path", "error in"=w9, "PreProc_Options_in"=w13, "Evaluation Metrics"=w4, "NNPC_in"=w72) -> ("error out"=w11:errorcluster, "NNPC_Paths"=w49:T1, "NNPC_out"=w41:T31)  [unwired: 4 in]
  "Model Paths" <- w49
  n21 = Build Array(w3) -> (w5:T29[])
  n22 = call <vilib>:"NNPC_Destroy.vi"("Datasets_to_Destroy"=w5, "error in"=w11, "NNPC_in"=w41) -> ("error out"=w8:errorcluster)  [unwired: 8 in]
  n23 = call "NN_Get_T_dT.vim"("T_in"=w89, "error in"=w8) -> ("error out"=w7:errorcluster, "dT"=→"dT_Total":dbl)  [unwired: 5 in, 1 out]
  n24 = call "Separate_Detections_into_Good_and_Bad.vi"("Dataset"=w2, "error in"=w7, "Pixel Scores"=w65, "Image Scores"=w66) -> ("error out"=w6:errorcluster, "Bad Samples"=w62:T23[], "Good Samples"=w61:T23[])  [unwired: 5 in]
  n25 = Unbundle By Name(w49) -> ("CFG"=w51:path)
  n26 = case shown="True" w68 {
    tunnel: w51 -> [_ w108]
    tunnel: [w104 w107] -> w31
    tunnel: w6 -> [w104 w106]
    frame False {
    }
    frame True {
      n27 = control-ref of="This VI"() -> (w118:refnum<vi>)
      n28 = call <vilib>:"Get File Extension.vi"("error in (no error)"=w106, "file"=w108) -> ("error out"=w105:errorcluster, "filename without extension"=w113:string)  [unwired: 5 in, 3 out]
      n29 = Strip Path(path=w108) -> (stripped path=w110:path)  [unwired: 1 out]
      n30 = invoke class="VI" method="FP.Get Image"(reference=w118, error in=w105, "visible area only"=FALSE ("Visible Area Only"), "image depth"=24 ("Image Depth")) -> (error out=w114:errorcluster, "image data"=w115:T48)  [unwired: 2 in, 4 out]
      n31 = Concatenate Strings(w113, ".png" ("string")) -> (w111:string)
      n32 = Build Path(base path=w110, name or relative path=w111) -> (appended path=w109:path)
      n33 = call <vilib>:"Write PNG File.vi"("error in (no error)"=w114, "image data"=w115, "path to PNG file"=w109) -> ("error out"=w107:errorcluster)  [unwired: 7 in, 1 out]
    }
  }
  n34 = Unbundle By Name(w41) -> ("NN.NN_Device"=w39:T4)
  n35 = Bundle By Name(cluster=T2 {"Input_Dims"={"C"=-1, "H"=-1, "W"=-1}, "mBatch"=1, "Device"=enum."GPU", "GPU Id"=0} ("NNPC_Setup"), "Device"=w39) -> (w40:T2)
  n36 = call <vilib>:"NNPC_Init(Inference).vi"("error in"=w31, "NNPC_Setup"=w40, "NNPC_Paths"=w49) -> ("error out"=w30:errorcluster, "PreProc_Options"=w12:T25, "NNPC_out"=w22:T31)  [unwired: 4 in, 2 out]
  n37 = call <vilib>:"NNPC_Read_Eval_Results.vi"("error in (no error)"=w30, "CFG file path"=w51) -> ("error out"=w23:errorcluster, "Evaluation_Results"=w50:T49)  [unwired: 8 in]
  n38 = Unbundle By Name(w22) -> ("NN"=w20:T32)
  n39 = call "Calculate_NXY_Coords_and_Dim_Info_of_Selected_Coreset_Indices.vi"("error in (no error)"=w23, "Selected_Feature_Coords"=w16, "NNPC_Instance"=w22) -> ("error out"=w24:errorcluster, "Selected_Coreset_Element_Info"=w25:T50)  [unwired: 7 in]
  n40 = call <vilib>:"NN_Get_Layer(Last).vi"("error in (no error)"=w24, "NN in"=w20) -> ("error out"=w21:errorcluster, "Last_Layer"=w27:T52)  [unwired: 6 in, 2 out]
  n41 = call "IMAQ Create"("Image Name"="closest_sample", "Image Type"=w36, "error in (no error)"=w21) -> ("New Image"=w33:T17, "error out"=w34:errorcluster)  [unwired: 2 in]
  n42 = Unbundle By Name(w3) -> ("Dataset_Size"=→"Dataset Size":i32, "File Paths"=w18:path[])
  n43 = local read "DS Selector"() -> (w63:enum16{"Good", "Bad", "Both"})
  n44 = property on="DS Selector" class="Enum (strict)"(error in=w34, "Val(Sgnl)"=w63) -> (error out=w43:errorcluster)  [unwired: 1 in, 1 out]
  n45 = Unbundle By Name(w27) -> ("RecptField.Dims.V"=w26:i32)
  n46 = while {
    tunnel: "Ground_Truth_Folder_Path" -> [w141]
    tunnel: w61 -> [w140]
    tunnel: w62 -> [w139]
    shift-right: [w138] -> _
    shift-left: T23[] [] ("Bad Samples") -> [w137]
    tunnel: w12 -> [w135]
    tunnel: w50 -> [w134]
    tunnel: w22 -> [w133]
    tunnel: w26 -> [w132]
    tunnel: w25 -> [w131]
    tunnel: w18 -> [w130]
    tunnel: [w129] -> w19
    shift-right: [w128] -> _
    shift-left: w37 -> [w127]
    shift-right: [w124] -> _
    shift-left: T17[] [] ("Anomaly Detection Rresults") -> [w123]
    tunnel: w33 -> [w121]
    tunnel: w43 -> [w142]
    tunnel: [w126] -> w17
    stop <- w136 stop-if-true
    n47 = event shown="[1] Timeout" {
      selector: _ -> [_ _ _ _ _]
      dyn-events: _ -> [_ _ _ _ _]
      timeout: 100 -> [_ _ _ _ _]
      tunnel: w142 -> [w180 w264 w323 w329 w345]
      tunnel: [w161 w230 w322 w328 w343] -> w126
      tunnel: w141 -> [w181 _ _ _ _]
      tunnel: w140 -> [_ _ _ w333 _]
      tunnel: w139 -> [_ _ _ w332 _]
      tunnel: [w167 w289 w320 w331 w350] -> w138
      tunnel: w137 -> [w167 w289 w320 _ w352]
      tunnel: w135 -> [w168 w219 _ _ _]
      tunnel: w134 -> [w149 _ _ _ _]
      tunnel: w133 -> [w162 w288 w318 w325 w341]
      tunnel: w132 -> [_ w270 _ _ _]
      tunnel: w131 -> [_ w239 _ _ _]
      tunnel: w130 -> [_ w269 _ _ _]
      tunnel: [w164 w288 w318 w325 w341] -> w129
      tunnel: [w163 w267 w321 w327 w342] -> w128
      tunnel: w127 -> [_ w267 w321 w327 w342]
      tunnel: w123 -> [_ w266 w319 w326 w340]
      tunnel: [_ "Stop" _ _ _] -> w125
      tunnel: [w146 w266 w319 w326 w340] -> w124
      tunnel: w121 -> [_ w265 _ _ _]
      tunnel: "UpScale Factor" -> [w155 w221 _ _ _]
      tunnel: "Pixel_Thrshld(Custom)" -> [w154 w240 _ _ _]
      tunnel: [w143 _ _ _ _] -> _
      tunnel: [w144 _ _ _ _] -> _
      event "index", "Image_Thrshld(Custom)", "Pixel_Thrshld(Custom)", "UpScale Factor": Value Change {
        n48 = event-data() -> ()  [unwired: 1 in, 6 out]
        n49 = Index Array(array=w167, index="index") -> (element=w179:T23)
        n50 = Unbundle By Name(w179) -> ("File Path"=w158:path)
        "Image_File_Path" <- w158
        n51 = call "Find_GT_File_Path.vi"("error in"=w180, "GT Mask Folder Path"=w181, "Image File Path"=w158) -> ("error out"=w176:errorcluster, "GT File Path"=w184:path, "Image File Path out"=w177:path)  [unwired: 5 in, 1 out]
        n52 = Bundle By Name(cluster=T60 {"ROI_Options"={"Color"=16717824, "Width"=3, "Drawing Mode"=enum."Frame"}, "Heatmap_Options"={"ColorMap"=enum."Jet", "Alpha"=0.4, "Heatmap Range"={"Min"=0.089999996, "Max"=0.18}}, "Report_Images_CFG"={"Original Image"=TRUE, "Ground Truth"=TRUE, "HeatMap"=TRUE, "Mask"=TRUE, "Segmentation"=TRUE}} ("Display_Options"), "Heatmap_Options.Heatmap Range"="Heatmap Range", "ROI_Options.Color"="ROI Color") -> (w152:T60)
        n53 = Unbundle By Name(w162) -> ("NN.NN_Device"=w165:T4)
        n54 = call "Read_Image.vi"("PreProcessing_Options"=w168, "error in"=w176, "Img Path"=w177) -> ("error out"=w174:errorcluster, "Image Out(Cropped)"=w156:T17, "Image Out (Preproc)"=w157:sgl[][][])  [unwired: 3 in, 3 out]
        n55 = call-poly <vilib>:"NNPC_Predict.vi"("Feature_Scorer_Params"=T21 {"Nearest_Neighbors"=1, "Calculate Anomaly Map"=TRUE, "Gaussian_Blur"={"Kernel_Size"=33, "Sigma"=4.0}}, "error in"=w174, "Image_in"=w157, "NNPC_in"=w162) -> ("error out"=w170:errorcluster, "Anomaly_Map"=w172:sgl[][], "Pred_Score"=w171:sgl, "NNPC_out"=w164:T31, "Distance_Matrix"=w169:variant, "dT_Predict"=w160:dbl)  [unwired: 2 in]
        "Img_Score" <- w171
        n56 = call "Combine_Anomaly_Detection_Results.vi"("Relative Resolution"=w155, "Evaluation_Results"=w149, "Display_Options"=w152, "Pixel Anomaly Thrshld"=w154, "error in"=w170, "Anomaly Map"=w172, "Gt File Path"=w184, "Orig Image In"=w156) -> ("error out"=w166:errorcluster, "Anomaly Detection Results"=w145:T65)  [unwired: 1 in, 1 out]
        n57 = call <vilib>:"Mean PtByPt.vi"("x"=w160) -> ("mean"=→"dT_Predict":dbl)  [unwired: 3 in, 1 out]
        n58 = Cluster To Array(cluster=w145) -> (array=w146:T17[])
        n59 = Unbundle By Name(w149) -> ("Threshold(Image)"=w148:sgl, "Threshold(Pixel)"=→"Pixel_Thrshld (Eval)":sgl)
        "Image_Thrshld (Eval)" <- w148
        n60 = Unbundle By Name(w145) -> ("Image"=w143:T17, "Predicted Mask"=w144:T17)
        n61 = case shown="\"GPU\"" w165 {
          tunnel: [w189 w197] -> w163
          tunnel: [w187 w196] -> w161
          tunnel: w169 -> [w192 w195]
          tunnel: w166 -> [w191 w194]
          frame "CPU", Default {
            n62 = Variant To Data(error in=w191, type=refnum<data-value> refnum ("data value reference"), Variant=w192) -> (data=w190:refnum<data-value>, error out=w188:errorcluster)
            n63 = call-poly <vilib>:"NN_Data_Get_ValByRef.vi"("error in (no error)"=w188, "DVR(2D_SGL)"=w190) -> ("error out"=w187:errorcluster, "Value(2D_SGL)"=w189:sgl[][])  [unwired: 6 in]
          }
          frame "GPU" {
            n64 = disable-structure shown="USE_CULAB==TRUE" {
              disable-tunnel: [w204 _] -> w197
              disable-tunnel: [w200 w205] -> w196
              disable-tunnel: w195 -> [w199 _]
              disable-tunnel: w194 -> [w198 w206]
              frame condition #0 (active) {
                n65 = Variant To Data(error in=w198, type=refnum<class "T2D_SGL.lvclass"> refnum ("Features"), Variant=w199) -> (data=w202:refnum<class "T2D_SGL.lvclass">, error out=w201:errorcluster)
                n66 = call-poly <vilib>:"CU_Tensor_Pull.vi"("error in (no error)"=w201, "T2D_SGL in"=w202) -> ("2D_SGL_Data"=w204:sgl[][], "error out"=w200:errorcluster)  [unwired: 7 in, 1 out]
              }
              frame condition #1 {
                n67 = Build Array("In order to use GPU for Patchcore, please install CuLab Toolkit and create and set conditional disable variable  with name  \"USE_CULAB\" with value \"TRUE\"." ("Message")) -> (w210:string[])
                n68 = call <vilib>:"NN_Generate_Custom_Error.vi"("show call chain? (TRUE)"=TRUE ("show call chain? (False)"), "error in (no error)"=w206, "Message"=w210, "Error_code"=403665) -> ("error out"=w205:errorcluster)  [unwired: 7 in]
              }
            }
          }
        }
        n69 = Less Than 0?(x="Image_Thrshld(Custom)") -> (x < 0?=w186:bool)
        n70 = Array Max & Min(array=w172) -> (max value=→"Pixel_Score(Max)":sgl)  [unwired: 3 out]
        n71 = Select(t=w148, s=w186, f="Image_Thrshld(Custom)") -> (s? t:f=w185:sgl)
        n72 = Greater?(x=w171, y=w185) -> (0:→"Anomaly?":bool)
      }
      event Timeout {
        w216 = u32 1 items=["Zero Order", "Bi-Linear", "Quadratic", "Cubic Spline"] ("Interpolation Type")
        n73 = event-data() -> ()  [unwired: 1 in, 1 out]
        n74 = local read "Last Mouse Position:All Elements"() -> (w273:cluster{"X":i32, "Y":i32})
        n75 = property on="Anomaly Detection Result" class="ImageControl"() -> ("Last Mouse Position"=w281:cluster{"X":i32, "Y":i32})  [unwired: 2 in, 2 out]
        n76 = Index Array(array=w266, index="Display_Image") -> (element=w259:T17)
        n77 = Select(t=w281, s="Search Mode", f=w273) -> (s? t:f=w258:cluster{"X":i32, "Y":i32})
        n78 = Divide(x=w258, y=w221) -> (x/y=w255:cluster{"X":sgl, "Y":sgl})
        n79 = To Long Integer(number=w255) -> (32bit integer=w253:cluster{"X":i32, "Y":i32})
        n80 = call "Pixel_Coords_To_Patch_Index.vi"("Selected_Coreset_Element_Info"=w239, "Coords"=w253) -> ("Flat_Patch_Coords"=w282:i32)  [unwired: 9 in]
        n81 = Index Array(array=w267, index (row)=w282) -> (element=w274:sgl[])  [unwired: 1 in]
        n82 = call "Find_Closeest_Embedding_Idx.vi"("Selected_Coreset_Element_Info"=w239, "Pixel_Thrshld(Custom)"=w240, "Distance_From_Embedding"=w274) -> ("Closest_Samples"=w283:T66[])  [unwired: 8 in]
        n83 = Array Size(array=w283) -> (size(s)=w284:i32)
        "#Closest_Samples" <- w284
        n84 = Decrement(x=w284) -> (x-1=w286:i32)
        n85 = property on="Closest_Idx" class="DigNum (strict)"("Maximum"=w286, "Minimum"=0.0 ("Data Entry Limits:Minimum")) -> ()  [unwired: 2 in, 2 out]
        n86 = Index Array(array=w283, index="Closest_Idx") -> (element=w248:T66)
        n87 = Unbundle By Name(w248) -> ("Feature_Coords"=w247:T47, "Score"=→"Closest_Score":sgl)
        n88 = Unbundle By Name("ROI Scales") -> ("Patch"=w275:sgl, "Receptive_Field"=w225:sgl)
        n89 = call "IMAQ Clear Overlay"("error in (no error)"=w264, "Image"=w259) -> ("error out"=w224:errorcluster, "Image Out"=w217:T17)  [unwired: 8 in]
        n90 = Unbundle By Name(w247) -> ("Idx"=w254:i32, "i"=w245:i32, "j"=w244:i32)
        n91 = Unbundle By Name(w219) -> ("Cropping"=w226:T26)
        n92 = Index Array(array=w269, index=w254) -> (element=w263:path)
        "Closest_Train_File_Path" <- w263
        n93 = Unbundle By Name(w253) -> ("Y"=w262:i32, "X"=w261:i32)
        n94 = Unbundle By Name(w239) -> ("Stride"=w222:i32)
        n95 = Bundle By Name(cluster=T51 {"H"=0, "W"=0} ("Coords_In"), "H"=w245, "W"=w244) -> (w243:T51)
        n96 = call "IMAQ ReadFile"("File Path"=w263, "error in (no error)"=w224, "Image"=w265) -> ("error out"=w229:errorcluster, "Image Out"=w227:T17)  [unwired: 4 in, 3 out]
        n97 = Bundle By Name(cluster=T51 {"H"=0, "W"=0} ("Coords_Out"), "H"=w262, "W"=w261) -> (w251:T51)
        n98 = call "Img_Center_Crop.vi"("Crop_CFG"=w226, "error in"=w229, "Image Dest In"=w227, "Image Src In"=w227) -> ("error out"=w212:errorcluster, "Image Dest Out"=w215:T17)  [unwired: 6 in]
        n99 = Multiply(x=w270, y=w225) -> (x*y=w279:sgl)
        n100 = call "Coerce_and_Center_Coords.vi"("Coords_In"=w251, "Feature_Size"=w222) -> ("Coords_Out"=w250:T51)  [unwired: 5 in]
        n101 = call "Coerce_and_Center_Coords.vi"("Coords_In"=w243, "Feature_Size"=w222) -> ("Coords_Out"=w242:T51)  [unwired: 5 in]
        n102 = Multiply(x=w222, y=w275) -> (x*y=w280:sgl)
        n103 = call "IMAQ GetImageSize"("Image"=w217, "error in (no error)"=w212) -> ("Y Resolution"=w214:i32, "X Resolution"=w213:i32, "error out"=w211:errorcluster)  [unwired: 2 in]
        n104 = Build Array(w280, w279) -> (w277:sgl[])
        n105 = call "IMAQ Resample"("X Resolution"=w213, "Y Resolution"=w214, "error in (no error)"=w211, "Interpolation Type"=w216, "Image Src"=w215) -> ("error out"=w228:errorcluster, "Image Dst Out"=w218:T17)  [unwired: 5 in]
        n106 = Multiply(x=w222, y=w221) -> (x*y=w220:sgl)
        n107 = call "Pixel_Coords_to_Feature_Coords(SS).vi"("Frame_Dims"=w277, "Center_Coords"=w250) -> ("Frames"=w278:T67[])  [unwired: 9 in]
        n108 = call "Pixel_Coords_to_Feature_Coords(SS).vi"("Frame_Dims"=w277, "Center_Coords"=w242) -> ("Frames"=w285:T67[])  [unwired: 9 in]
        n109 = case shown="True" "Show Patch Grid?" {
          tunnel: w217 -> [w292 w303]
          tunnel: [w292 w302] -> w238
          tunnel: w224 -> [w291 w301]
          tunnel: w220 -> [_ w300]
          tunnel: w218 -> [w293 w299]
          tunnel: [w293 w298] -> w233
          tunnel: [w290 w295] -> w237
          tunnel: w228 -> [w290 w297]
          tunnel: [w291 w294] -> w234
          frame False {
          }
          frame True {
            w296 = u32 6618880 ("Grid Color")
            n110 = call "Draw_Grid.vi"("Grid Color"=w296, "error in (no error)"=w301, "Grid_Size"=w300, "Image_In"=w303) -> ("error out"=w294:errorcluster, "Image_Out"=w302:T17)  [unwired: 6 in]
            n111 = call "Draw_Grid.vi"("Grid Color"=w296, "error in (no error)"=w297, "Grid_Size"=w300, "Image_In"=w299) -> ("error out"=w295:errorcluster, "Image_Out"=w298:T17)  [unwired: 6 in]
          }
        }
        n112 = Multiply(x=w278, y=w221) -> (x*y=w256:T67[])
        n113 = Multiply(x=w285, y=w221) -> (x*y=w257:T67[])
        n114 = for {
          tunnel: "Feature Color" -> [w310]
          tunnel: w256 -> [w309] mode=indexing
          tunnel: w234 -> [w308]
          shift-right: [w306] -> w236
          shift-left: w238 -> [w307]
          tunnel: [w304] -> w232
          stop <- w304 stop-if-true
          w305 = u32 0 items=["Frame", "Fill"] ("Drawing Mode (Frame)")
          n115 = call "IMAQ Overlay Rectangle"("Color"=w310, "error in (no error)"=w308, "Drawing Mode (Frame)"=w305, "Rectangle"=w309, "Image"=w307) -> ("error out"=w304:errorcluster, "Image Out"=w306:T17)  [unwired: 5 in]
        }
        "Anomaly Detection Result" <- w236
        n116 = for {
          tunnel: "Feature Color" -> [w317]
          tunnel: w257 -> [w316] mode=indexing
          shift-right: [w313] -> w235
          shift-left: w233 -> [w315]
          tunnel: w237 -> [w314]
          tunnel: [w311] -> w231
          stop <- w311 stop-if-true
          w312 = u32 0 items=["Frame", "Fill"] ("Drawing Mode (Frame)")
          n117 = call "IMAQ Overlay Rectangle"("Color"=w317, "error in (no error)"=w314, "Drawing Mode (Frame)"=w312, "Rectangle"=w316, "Image"=w315) -> ("error out"=w311:errorcluster, "Image Out"=w313:T17)  [unwired: 5 in]
        }
        "Closest_Train_Sample" <- w235
        n118 = Merge Errors(w232, w231) -> (w230:errorcluster)
      }
      event "Anomaly Detection Result": Mouse Down {
        n119 = event-data() -> ()  [unwired: 1 in, 1 out]
        n120 = property on="Anomaly Detection Result" class="ImageControl"(error in=w323) -> (error out=w322:errorcluster, "Last Mouse Position"=→"Last Mouse Position:All Elements":cluster{"X":i32, "Y":i32})  [unwired: 1 in, 1 out]
      }
      event "DS Selector": Value Change {
        n121 = event-data() -> ("NewVal"=w334:enum16{"Good", "Bad", "Both"})  [unwired: 1 in]
        n122 = local read "Order"() -> (w330:enum16{"Ascending", "Descending", "File"})
        n123 = case shown="\"Good\", Default" w334 {
          tunnel: w333 -> [w335 _ w339]
          tunnel: w332 -> [_ w336 w338]
          tunnel: [w335 w336 w337] -> w331
          frame "Good", Default {
          }
          frame "Bad" {
          }
          frame "Both" {
            n124 = Build Array (concatenate)(w339, w338) -> (w337:T23[])
          }
        }
        n125 = property on="Order" class="Enum (strict)"(error in=w329, "Val(Sgnl)"=w330) -> (error out=w328:errorcluster)  [unwired: 1 in, 1 out]
      }
      event "Order": Value Change {
        w348 = u32 0 ("Data Entry Limits:Minimum")
        n126 = event-data() -> ("NewVal"=w353:enum16{"Ascending", "Descending", "File"})  [unwired: 1 in]
        n127 = case shown="\"Ascending\", Default" w353 {
          tunnel: [w354 w370 w383] -> w350
          tunnel: w352 -> [w356 w369 w383]
          frame "Ascending", Default {
            n128 = for {
              tunnel: w356 -> [w365] mode=indexing
              tunnel: [w364] -> w358 mode=indexing
              i -> [w363]
              n129 = Unbundle By Name(w365) -> ("Image Score"=w362:sgl)
              n130 = Bundle("Image Score"=w362, w363) -> (w364:cluster{"Image Score":sgl, i32})  [unwired: 1 in]
            }
            n131 = Sort 1D Array(array=w358) -> (sorted array=w357:cluster{"Image Score":sgl, i32}[])
            n132 = for {
              tunnel: w357 -> [w367] mode=indexing
              tunnel: [w366] -> w355 mode=indexing
              n133 = Unbundle(w367) -> (w366:i32)  [unwired: 1 out]
            }
            n134 = for {
              tunnel: w356 -> [w361]
              tunnel: w355 -> [w360] mode=indexing
              tunnel: [w359] -> w354 mode=indexing
              n135 = Index Array(array=w361, index=w360) -> (element=w359:T23)
            }
          }
          frame "Descending" {
            n136 = for {
              tunnel: w369 -> [w380] mode=indexing
              tunnel: [w379] -> w371 mode=indexing
              i -> [w378]
              n137 = Unbundle By Name(w380) -> ("Image Score"=w377:sgl)
              n138 = Bundle("Image Score"=w377, w378) -> (w379:cluster{"Image Score":sgl, i32})  [unwired: 1 in]
            }
            n139 = Sort 1D Array(array=w371) -> (sorted array=w372:cluster{"Image Score":sgl, i32}[])
            n140 = Reverse 1D Array(array=w372) -> (reversed array=w368:cluster{"Image Score":sgl, i32}[])
            n141 = for {
              tunnel: w368 -> [w382] mode=indexing
              tunnel: [w381] -> w373 mode=indexing
              n142 = Unbundle(w382) -> (w381:i32)  [unwired: 1 out]
            }
            n143 = for {
              tunnel: w369 -> [w376]
              tunnel: w373 -> [w375] mode=indexing
              tunnel: [w374] -> w370 mode=indexing
              n144 = Index Array(array=w376, index=w375) -> (element=w374:T23)
            }
          }
          frame "File" {
          }
        }
        n145 = local read "index"() -> (w346:i32)
        n146 = property on="index" class="DigNum (strict)"(error in=w345, "Val(Sgnl)"=w346) -> (error out=w344:errorcluster)  [unwired: 1 in, 1 out]
        n147 = Array Size(array=w350) -> (size(s)=w349:i32)
        n148 = Decrement(x=w349) -> (x-1=w351:i32)
        n149 = property on="index" class="DigNum (strict)"(error in=w344, "Maximum"=w351, "Minimum"=w348, "OutOfRngActMax"=u8 1 ("Response to Value Outside Limits:Maximum"), "OutOfRngActMin"=w348) -> (error out=w343:errorcluster)  [unwired: 1 in, 1 out]
      }
    }
    n150 = Or(x=w125, y=w126) -> (x .or. y?=w136:bool)
  }
  n151 = Build Array(w2) -> (w1:T29[])
  n152 = call <vilib>:"NNPC_Destroy.vi"("Datasets_to_Destroy"=w1, "error in"=w17, "NNPC_in"=w19) -> ("error out"=→"error out":errorcluster)  [unwired: 8 in]
